vi "Validate JSON structure (LabVIEW format).vi"(8 "error in (no error)":errorcluster, 9 "Reference cluster":variant, 10 "Compare structure":string="{\r\n    \"SpecificationVersion\":\"1\",\r\n    \"CompatibleSoftwareVersions\":[\r\n        \"1.0\"\r\n    ],\r\n    \"AlgoParameters\":{\r\n        \"PartsList\":[\r\n            {\r\n                \"Name\":\"TT-1478\",\r\n                \"ImageStreams\":[\r\n                    {\r\n                        \"ThreadName\":\"TopRack\",\r\n                        \"RackEnable\":true,\r\n                        \"ThreadId\":0,\r\n                        \"RackId\":0,\r\n                        \"DifferenceParameter\":0,\r\n                        \"SplitCameraIDs\":[\r\n                            0\r\n                        ],\r\n                        \"ImagingViews\":[\r\n                            {\r\n                                \"ViewName\":\"Top\",\r\n                                \"ViewEnable\":true,\r\n                                \"ImageID\":0,\r\n                                \"CameraID\":0,\r\n                                \"CalibrationFilePath\":\"Algorithm\\\\Calibration\\\\TT Top Calib\",\r\n                                \"CalibImageFormat\":\"png\",\r\n                                \"ReferenceCoordSystem\":{\r\n                                    \"Method\":{\r\n                                        \"Algo\":\"Detect Ellipses v2\",\r\n                                        \"BaseReference\":{\r\n                                            \"OriginX\":902,\r\n                                            \"OriginY\":425,\r\n                                            \"Angle\":0,\r\n                                            \"AxisReference\":0\r\n                                        }\r\n                                    },\r\n                                    \"ROI\":[\r\n                                        {\r\n                                            \"ROI\":{\r\n                                                \"Left\":820,\r\n                                                \"Top\":170,\r\n                                                \"Right\":1110,\r\n                                                \"Bottom\":630,\r\n                                                \"Rotation\":0\r\n                                            },\r\n                                            \"EdgeOptions\":{\r\n                                                \"EdgePolarity\":2,\r\n                                                \"KernelSize\":5,\r\n                                                \"Width\":5,\r\n                                                \"MinimumEdgeStrength\":50,\r\n                                                \"InterpolationType\":0,\r\n                                                \"DataProcessingMethod\":0\r\n                                            },\r\n                                            \"LineOptions\":{\r\n                                                \"NumberofLines\":1,\r\n                                                \"Type\":0,\r\n                                                \"MinScore\":10,\r\n                                                \"MaxScore\":1000,\r\n                                                \"Orientation\":0,\r\n                                                \"AngleRange\":60,\r\n                                                \"AngleTolerance\":10,\r\n                                                \"StepSize\":15,\r\n                                                \"MinSNR\":10,\r\n                                                \"MinPoints\":25,\r\n                                                \"HoughIterations\":5\r\n                                            },\r\n                                            \"Process\":0,\r\n                                            \"StepSize\":10,\r\n                                            \"SearchDirection\":1,\r\n                                            \"CircleEdgeOptions\":{\r\n                                                \"SearchDirection\":1,\r\n                                                \"EdgeOptions\":{\r\n                                                    \"EdgePolarity\":0,\r\n                                                    \"KernelSize\":7,\r\n                                                    \"Width\":5,\r\n                                                    \"MinimumEdgeStrength\":50,\r\n                                                    \"InterpolationType\":0,\r\n                                                    \"DataProcessingMethod\":0\r\n                                                }\r\n                                            },\r\n                                            \"CircleFitOptions\":{\r\n                                                \"Process\":3,\r\n                                                \"StepSize\":3,\r\n                                                \"MAxPixelRadius\":3\r\n                                            },\r\n                                            \"CircleSearchDirection\":1,\r\n                                            \"CurveParameters\":{\r\n                                                \"ExtractionMode\":0,\r\n                                                \"EdgeThreshold\":50,\r\n                                                \"EdgeFilterSize\":0,\r\n                                                \"MinLength\":25,\r\n                                                \"RowSearchStepSize\":15,\r\n                                                \"ColSearchStepSize\":15,\r\n                                                \"MaxEndpointGap\":10,\r\n                                                \"Closed\":true,\r\n                                                \"Subpixel\":true\r\n                                            },\r\n                                            \"MinimumMatchScore\":800,\r\n                                            \"CircleDescriptor\":{\r\n                                                \"MinRadius\":3,\r\n                                                \"MaxRadius\":200\r\n                                            },\r\n                                            \"EllipseDescriptor\":{\r\n                                                \"MinMajorRadius\":3,\r\n                                                \"MaxMajorRadius\":200,\r\n                                                \"MinMinorRadius\":3,\r\n                                                \"MaxMinorRadius\":100\r\n                                            },\r\n                                            \"ParallelLines\":{\r\n                                                \"First\":30,\r\n                                                \"Second\":45,\r\n                                                \"Third\":60\r\n                                            }\r\n                                        }\r\n                                    ],\r\n                                    \"Name\":\"FirstReference\",\r\n                                    \"OverlayOptions\":{\r\n                                        \"OverlayEnable\":true,\r\n                                        \"OverlayText\":\"Height\",\r\n                                        \"OverlayCoords\":[\r\n                                            5,\r\n                                            8\r\n                                        ],\r\n                                        \"OverlayAngle\":56,\r\n                                        \"OverlayTextSize\":6,\r\n                                        \"OverlayTextColor\":\"Blue\",\r\n                                        \"OverlayROI\":false,\r\n                                        \"OverlayRakeLine\":false,\r\n                                        \"OverlayPoints\":false\r\n                                    }\r\n                                },\r\n                                \"CameraAngle\":[\r\n                                    15\r\n                                ]\r\n                            }\r\n                        ]\r\n                    }\r\n                ],\r\n                \"Measurements\":[\r\n                    {\r\n                        \"RackID\":0,\r\n                        \"ImageID\":0,\r\n                        \"CameraID\":0,\r\n                        \"MeasurementId\":1,\r\n                        \"Name\":\"L\",\r\n                        \"AlgoName\":\"AET\",\r\n                        \"Type\":\"Max\",\r\n                        \"MeasurementEnable\":true,\r\n                        \"AlgorithmSequence\":{\r\n                            \"RefernceEdge\":{\r\n                                \"Enable\":true,\r\n                                \"Method\":\"LineFinding\",\r\n                                \"RefROI\":{\r\n                                    \"Left\":330,\r\n                                    \"Top\":200,\r\n                                    \"Right\":400,\r\n                                    \"Bottom\":500,\r\n                                    \"Rotation\":0\r\n                                },\r\n                                \"EdgeOptions\":{\r\n                                    \"EdgePoarity\":2,\r\n                                    \"KernelSize\":5,\r\n                                    \"Width\":5,\r\n                                    \"MinimumEdgeStrength\":50,\r\n                                    \"InterpolationType\":0,\r\n                                    \"DataProcessingMethod\":0\r\n                                },\r\n                                \"LineOptions\":{\r\n                                    \"NumberofLines\":1,\r\n                                    \"Type\":0,\r\n                                    \"MinScore\":10,\r\n                                    \"MaxScore\":1000,\r\n                                    \"Orientation\":5,\r\n                                    \"AngleRange\":70,\r\n                                    \"AngleTolerance\":1,\r\n                                    \"StepSize\":3,\r\n                                    \"MinSNR\":0,\r\n                                    \"MinPoints\":25,\r\n                                    \"HoughIterations\":5\r\n                                },\r\n                                \"SearchDirection\":2\r\n                            },\r\n                            \"Measurement\":{\r\n                                \"ROI1\":{\r\n                                    \"Enable\":true,\r\n                                    \"ROI\":{\r\n                                        \"Left\":320,\r\n                                        \"Top\":200,\r\n                                        \"Right\":330,\r\n                                        \"Bottom\":600,\r\n                                        \"Rotation\":0\r\n                                    },\r\n                                    \"EdgeOptions\":{\r\n                                        \"EdgePoarity\":0,\r\n                                        \"KernelSize\":5,\r\n                                        \"Width\":5,\r\n                                        \"MinimumEdgeStrength\":50,\r\n                                        \"InterpolationType\":0,\r\n                                        \"DataProcessingMethod\":0\r\n                                    },\r\n                                    \"LineOptions\":{\r\n                                        \"NumberofLines\":1,\r\n                                        \"Type\":1,\r\n                                        \"MinScore\":10,\r\n                                        \"MaxScore\":1000,\r\n                                        \"Orientation\":0,\r\n                                        \"AngleRange\":30,\r\n                                        \"AngleTolerance\":1,\r\n                                        \"StepSize\":3,\r\n                                        \"MinSNR\":0,\r\n                                        \"MinPoints\":25,\r\n                                        \"HoughIterations\":5\r\n                                    },\r\n                                    \"Process\":1,\r\n                                    \"StepSize\":3,\r\n                                    \"SearchDirection\":2,\r\n                                    \"CircleEdgeOptions\":{\r\n                                        \"SearchDirection\":0,\r\n                                        \"EdgeOptions\":{\r\n                                            \"EdgePoarity\":2,\r\n                                            \"KernelSize\":5,\r\n                                            \"Width\":5,\r\n                                            \"MinimumEdgeStrength\":50,\r\n                                            \"InterpolationType\":1,\r\n                                            \"DataProcessingMethod\":1\r\n                                        }\r\n                                    },\r\n                                    \"CircleFitOptions\":{\r\n                                        \"Process\":3,\r\n                                        \"StepSize\":3,\r\n                                        \"MAxPixelRadius\":3.8500000000000000000\r\n                                    },\r\n                                    \"CircleSearchDirection\":1,\r\n                                    \"CurveParameters\":{\r\n                                        \"ExtractionMode\":0,\r\n                                        \"EdgeThreshold\":50,\r\n                                        \"EdgeFilterSize\":0,\r\n                                        \"MinLength\":25,\r\n                                        \"RowSearchStepSize\":15,\r\n                                        \"ColSearchStepSize\":15,\r\n                                        \"MaxEndpointGap\":10,\r\n                                        \"Closed\":true,\r\n                                        \"Subpixel\":true\r\n                                    },\r\n                                    \"MinimumMatchScore\":800,\r\n                                    \"CircleDescriptor\":{\r\n                                        \"MinRadius\":3,\r\n                                        \"MaxRadius\":200\r\n                                    },\r\n                                    \"EllipseDescriptor\":{\r\n                                        \"MinMajorRadius\":2,\r\n                                        \"MaxMajorRadius\":200,\r\n                                        \"MinMinorRadius\":2,\r\n                                        \"MaxMinorRadius\":100\r\n                                    }\r\n                                },\r\n                                \"ROI2\":{\r\n                                    \"Enable\":false,\r\n                                    \"ROI\":{\r\n                                        \"Left\":739,\r\n                                        \"Top\":305,\r\n                                        \"Right\":763,\r\n                                        \"Bottom\":538,\r\n                                        \"Rotation\":0\r\n                                    },\r\n                                    \"EdgeOptions\":{\r\n                                        \"EdgePoarity\":0,\r\n                                        \"KernelSize\":5,\r\n                                        \"Width\":5,\r\n                                        \"MinimumEdgeStrength\":50,\r\n                                        \"InterpolationType\":0,\r\n                                        \"DataProcessingMethod\":0\r\n                                    },\r\n                                    \"LineOptions\":{\r\n                                        \"NumberofLines\":1,\r\n                                        \"Type\":1,\r\n                                        \"MinScore\":10,\r\n                                        \"MaxScore\":1000,\r\n                                        \"Orientation\":0,\r\n                                        \"AngleRange\":30,\r\n                                        \"AngleTolerance\":1,\r\n                                        \"StepSize\":3,\r\n                                        \"MinSNR\":0,\r\n                                        \"MinPoints\":25,\r\n                                        \"HoughIterations\":5\r\n                                    },\r\n                                    \"Process\":1,\r\n                                    \"StepSize\":2,\r\n                                    \"SearchDirection\":2,\r\n                                    \"CircleEdgeOptions\":{\r\n                                        \"SearchDirection\":0,\r\n                                        \"EdgeOptions\":{\r\n                                            \"EdgePoarity\":2,\r\n                                            \"KernelSize\":3,\r\n                                            \"Width\":3,\r\n                                            \"MinimumEdgeStrength\":50,\r\n                                            \"InterpolationType\":1,\r\n                                            \"DataProcessingMethod\":1\r\n                                        }\r\n                                    },\r\n                                    \"CircleFitOptions\":{\r\n                                        \"Process\":3,\r\n                                        \"StepSize\":3,\r\n                                        \"MAxPixelRadius\":3.8500000000000000000\r\n                                    },\r\n                                    \"CircleSearchDirection\":1,\r\n                                    \"CurveParameters\":{\r\n                                        \"ExtractionMode\":0,\r\n                                        \"EdgeThreshold\":50,\r\n                                        \"EdgeFilterSize\":0,\r\n                                        \"MinLength\":25,\r\n                                        \"RowSearchStepSize\":15,\r\n                                        \"ColSearchStepSize\":15,\r\n                                        \"MaxEndpointGap\":10,\r\n                                        \"Closed\":true,\r\n                                        \"Subpixel\":true\r\n                                    },\r\n                                    \"MinimumMatchScore\":800,\r\n                                    \"CircleDescriptor\":{\r\n                                        \"MinRadius\":3,\r\n                                        \"MaxRadius\":200\r\n                                    },\r\n                                    \"EllipseDescriptor\":{\r\n                                        \"MinMajorRadius\":2,\r\n                                        \"MaxMajorRadius\":200,\r\n                                        \"MinMinorRadius\":2,\r\n                                        \"MaxMinorRadius\":100\r\n                                    }\r\n                                }\r\n                            }\r\n                        },\r\n                        \"MathExpression\":{\r\n                            \"Algorithm\":\"Default\",\r\n                            \"MathExpression\":\"c = 1*c + 0\",\r\n                            \"ResultVariable\":\"c\"\r\n                        },\r\n                        \"MathCorrectionParameters\":{\r\n                            \"Radius\":1.1000000000000000000,\r\n                            \"CurlGap\":0.90000000000000000000,\r\n                            \"Thickness\":0.32000000000000000000,\r\n                            \"MeasurementIndices\":[\r\n                                1\r\n                            ],\r\n                            \"MathAlgoName\":\"Test\",\r\n                            \"MathAlgoFormula\":\"Test2\",\r\n                            \"CorrectionForAngle\":[\r\n                                -2\r\n                            ],\r\n                            \"NumericAray\":[\r\n                                1.1000000000000000000\r\n                            ],\r\n                            \"StringArray\":[\r\n                                \"Test\"\r\n                            ]\r\n                        },\r\n                        \"ResultVariableCluster\":{\r\n                            \"RVName\":\"c\",\r\n                            \"RVSequence\":\"MeasROI1\",\r\n                            \"RVIndex\":1,\r\n                            \"RVID\":1,\r\n                            \"RVValue\":22.600000000000000000\r\n                        },\r\n                        \"CalibrationCoefficients\":{\r\n                            \"A1\":1.6800000000000000000,\r\n                            \"A2\":1.7800000000000000000,\r\n                            \"A3\":1.7600000000000000000\r\n                        },\r\n                        \"UserCalibCoefficients\":{\r\n                            \"UserCorrectionLinearityCoeff\":0.80000000000000000000,\r\n                            \"UserCorrectionBiasCoeff\":0.44300000000000000000\r\n                        },\r\n                        \"SpecValues\":{\r\n                            \"LCL\":2.1500000000000000000,\r\n                            \"UCL\":2.3500000000000000000,\r\n                            \"LSL\":2.1500000000000000000,\r\n                            \"USL\":2.3500000000000000000,\r\n                            \"NominalValue\":2.2500000000000000000\r\n                        },\r\n                        \"OverlayOptions\":{\r\n                            \"OverlayEnable\":true,\r\n                            \"OverlayText\":\"Width\",\r\n                            \"OverlayCoords\":[\r\n                                5,\r\n                                8\r\n                            ],\r\n                            \"OverlayAngle\":56,\r\n                            \"OverlayTextSize\":6,\r\n                            \"OverlayTextColor\":\"Blue\",\r\n                            \"OverlayROI\":true,\r\n                            \"OverlayRakeLine\":true,\r\n                            \"OverlayPoints\":true\r\n                        },\r\n                        \"DatalogEnable\":true,\r\n                        \"DisplayIcon\":\"C:\\\\Desktop\\\\displayimage.png\"\r\n                    }\r\n                ]\r\n            },\r\n            {\r\n                \"Name\":\"Part 3\",\r\n                \"ImageStreams\":[\r\n                    {\r\n                        \"ThreadName\":\"TopRack3\",\r\n                        \"RackEnable\":true,\r\n                        \"ThreadId\":0,\r\n                        \"RackId\":0,\r\n                        \"DifferenceParameter\":0,\r\n                        \"SplitCameraIDs\":[\r\n                            0\r\n                        ],\r\n                        \"ImagingViews\":[\r\n                            {\r\n                                \"ViewName\":\"Top2\",\r\n                                \"ViewEnable\":true,\r\n                                \"ImageID\":0,\r\n                                \"CameraID\":0,\r\n                                \"CalibrationFilePath\":\"Algorithm\\\\Calibration\\\\TT Top Calib\",\r\n                                \"CalibImageFormat\":\"png\",\r\n                                \"ReferenceCoordSystem\":{\r\n                                    \"Method\":{\r\n                                        \"Algo\":\"Detect Ellipses v2\",\r\n                                        \"BaseReference\":{\r\n                                            \"OriginX\":902,\r\n                                            \"OriginY\":425,\r\n                                            \"Angle\":0,\r\n                                            \"AxisReference\":0\r\n                                        }\r\n                                    },\r\n                                    \"ROI\":[\r\n                                        {\r\n                                            \"ROI\":{\r\n                                                \"Left\":820,\r\n                                                \"Top\":170,\r\n                                                \"Right\":1110,\r\n                                                \"Bottom\":630,\r\n                                                \"Rotation\":0\r\n                                            },\r\n                                            \"EdgeOptions\":{\r\n                                                \"EdgePolarity\":2,\r\n                                                \"KernelSize\":5,\r\n                                                \"Width\":5,\r\n                                                \"MinimumEdgeStrength\":50,\r\n                                                \"InterpolationType\":0,\r\n                                                \"DataProcessingMethod\":0\r\n                                            },\r\n                                            \"LineOptions\":{\r\n                                                \"NumberofLines\":1,\r\n                                                \"Type\":0,\r\n                                                \"MinScore\":10,\r\n                                                \"MaxScore\":1000,\r\n                                                \"Orientation\":0,\r\n                                                \"AngleRange\":60,\r\n                                                \"AngleTolerance\":10,\r\n                                                \"StepSize\":15,\r\n                                                \"MinSNR\":10,\r\n                                                \"MinPoints\":25,\r\n                                                \"HoughIterations\":5\r\n                                            },\r\n                                            \"Process\":0,\r\n                                            \"StepSize\":10,\r\n                                            \"SearchDirection\":1,\r\n                                            \"CircleEdgeOptions\":{\r\n                                                \"SearchDirection\":1,\r\n                                                \"EdgeOptions\":{\r\n                                                    \"EdgePolarity\":0,\r\n                                                    \"KernelSize\":7,\r\n                                                    \"Width\":5,\r\n                                                    \"MinimumEdgeStrength\":50,\r\n                                                    \"InterpolationType\":0,\r\n                                                    \"DataProcessingMethod\":0\r\n                                                }\r\n                                            },\r\n                                            \"CircleFitOptions\":{\r\n                                                \"Process\":3,\r\n                                                \"StepSize\":3,\r\n                                                \"MAxPixelRadius\":3\r\n                                            },\r\n                                            \"CircleSearchDirection\":1,\r\n                                            \"CurveParameters\":{\r\n                                                \"ExtractionMode\":0,\r\n                                                \"EdgeThreshold\":50,\r\n                                                \"EdgeFilterSize\":0,\r\n                                                \"MinLength\":25,\r\n                                                \"RowSearchStepSize\":15,\r\n                                                \"ColSearchStepSize\":15,\r\n                                                \"MaxEndpointGap\":10,\r\n                                                \"Closed\":true,\r\n                                                \"Subpixel\":true\r\n                                            },\r\n                                            \"MinimumMatchScore\":800,\r\n                                            \"CircleDescriptor\":{\r\n                                                \"MinRadius\":3,\r\n                                                \"MaxRadius\":200\r\n                                            },\r\n                                            \"EllipseDescriptor\":{\r\n                                                \"MinMajorRadius\":3,\r\n                                                \"MaxMajorRadius\":200,\r\n                                                \"MinMinorRadius\":3,\r\n                                                \"MaxMinorRadius\":100\r\n                                            },\r\n                                            \"ParallelLines\":{\r\n                                                \"First\":30,\r\n                                                \"Second\":45,\r\n                                                \"Third\":60\r\n                                            }\r\n                                        }\r\n                                    ],\r\n                                    \"Name\":\"FirstReference\",\r\n                                    \"OverlayOptions\":{\r\n                                        \"OverlayEnable\":true,\r\n                                        \"OverlayText\":\"Height\",\r\n                                        \"OverlayCoords\":[\r\n                                            5,\r\n                                            8\r\n                                        ],\r\n                                        \"OverlayAngle\":56,\r\n                                        \"OverlayTextSize\":6,\r\n                                        \"OverlayTextColor\":\"Blue\",\r\n                                        \"OverlayROI\":false,\r\n                                        \"OverlayRakeLine\":false,\r\n                                        \"OverlayPoints\":false\r\n                                    }\r\n                                },\r\n                                \"CameraAngle\":[\r\n                                    15\r\n                                ]\r\n                            }\r\n                        ]\r\n                    }\r\n                ],\r\n                \"Measurements\":[\r\n                    {\r\n                        \"RackID\":0,\r\n                        \"ImageID\":0,\r\n                        \"CameraID\":0,\r\n                        \"MeasurementId\":2,\r\n                        \"Name\":\"Measurement 2\",\r\n                        \"AlgoName\":\"AET\",\r\n                        \"Type\":\"Max\",\r\n                        \"MeasurementEnable\":true,\r\n                        \"AlgorithmSequence\":{\r\n                            \"RefernceEdge\":{\r\n                                \"Enable\":true,\r\n                                \"Method\":\"LineFinding\",\r\n                                \"RefROI\":{\r\n                                    \"Left\":330,\r\n                                    \"Top\":200,\r\n                                    \"Right\":400,\r\n                                    \"Bottom\":500,\r\n                                    \"Rotation\":0\r\n                                },\r\n                                \"EdgeOptions\":{\r\n                                    \"EdgePoarity\":2,\r\n                                    \"KernelSize\":5,\r\n                                    \"Width\":5,\r\n                                    \"MinimumEdgeStrength\":50,\r\n                                    \"InterpolationType\":0,\r\n                                    \"DataProcessingMethod\":0\r\n                                },\r\n                                \"LineOptions\":{\r\n                                    \"NumberofLines\":1,\r\n                                    \"Type\":0,\r\n                                    \"MinScore\":10,\r\n                                    \"MaxScore\":1000,\r\n                                    \"Orientation\":5,\r\n                                    \"AngleRange\":70,\r\n                                    \"AngleTolerance\":1,\r\n                                    \"StepSize\":3,\r\n                                    \"MinSNR\":0,\r\n                                    \"MinPoints\":25,\r\n                                    \"HoughIterations\":5\r\n                                },\r\n                                \"SearchDirection\":2\r\n                            },\r\n                            \"Measurement\":{\r\n                                \"ROI1\":{\r\n                                    \"Enable\":true,\r\n                                    \"ROI\":{\r\n                                        \"Left\":320,\r\n                                        \"Top\":200,\r\n                                        \"Right\":330,\r\n                                        \"Bottom\":600,\r\n                                        \"Rotation\":0\r\n                                    },\r\n                                    \"EdgeOptions\":{\r\n                                        \"EdgePoarity\":0,\r\n                                        \"KernelSize\":5,\r\n                                        \"Width\":5,\r\n                                        \"MinimumEdgeStrength\":50,\r\n                                        \"InterpolationType\":0,\r\n                                        \"DataProcessingMethod\":0\r\n                                    },\r\n                                    \"LineOptions\":{\r\n                                        \"NumberofLines\":1,\r\n                                        \"Type\":1,\r\n                                        \"MinScore\":10,\r\n                                        \"MaxScore\":1000,\r\n                                        \"Orientation\":0,\r\n                                        \"AngleRange\":30,\r\n                                        \"AngleTolerance\":1,\r\n                                        \"StepSize\":3,\r\n                                        \"MinSNR\":0,\r\n                                        \"MinPoints\":25,\r\n                                        \"HoughIterations\":5\r\n                                    },\r\n                                    \"Process\":1,\r\n                                    \"StepSize\":3,\r\n                                    \"SearchDirection\":2,\r\n                                    \"CircleEdgeOptions\":{\r\n                                        \"SearchDirection\":0,\r\n                                        \"EdgeOptions\":{\r\n                                            \"EdgePoarity\":2,\r\n                                            \"KernelSize\":5,\r\n                                            \"Width\":5,\r\n                                            \"MinimumEdgeStrength\":50,\r\n                                            \"InterpolationType\":1,\r\n                                            \"DataProcessingMethod\":1\r\n                                        }\r\n                                    },\r\n                                    \"CircleFitOptions\":{\r\n                                        \"Process\":3,\r\n                                        \"StepSize\":3,\r\n                                        \"MAxPixelRadius\":3.8500000000000000000\r\n                                    },\r\n                                    \"CircleSearchDirection\":1,\r\n                                    \"CurveParameters\":{\r\n                                        \"ExtractionMode\":0,\r\n                                        \"EdgeThreshold\":50,\r\n                                        \"EdgeFilterSize\":0,\r\n                                        \"MinLength\":25,\r\n                                        \"RowSearchStepSize\":15,\r\n                                        \"ColSearchStepSize\":15,\r\n                                        \"MaxEndpointGap\":10,\r\n                                        \"Closed\":true,\r\n                                        \"Subpixel\":true\r\n                                    },\r\n                                    \"MinimumMatchScore\":800,\r\n                                    \"CircleDescriptor\":{\r\n                                        \"MinRadius\":3,\r\n                                        \"MaxRadius\":200\r\n                                    },\r\n                                    \"EllipseDescriptor\":{\r\n                                        \"MinMajorRadius\":2,\r\n                                        \"MaxMajorRadius\":200,\r\n                                        \"MinMinorRadius\":2,\r\n                                        \"MaxMinorRadius\":100\r\n                                    }\r\n                                },\r\n                                \"ROI2\":{\r\n                                    \"Enable\":false,\r\n                                    \"ROI\":{\r\n                                        \"Left\":739,\r\n                                        \"Top\":305,\r\n                                        \"Right\":763,\r\n                                        \"Bottom\":538,\r\n                                        \"Rotation\":0\r\n                                    },\r\n                                    \"EdgeOptions\":{\r\n                                        \"EdgePoarity\":0,\r\n                                        \"KernelSize\":5,\r\n                                        \"Width\":5,\r\n                                        \"MinimumEdgeStrength\":50,\r\n                                        \"InterpolationType\":0,\r\n                                        \"DataProcessingMethod\":0\r\n                                    },\r\n                                    \"LineOptions\":{\r\n                                        \"NumberofLines\":1,\r\n                                        \"Type\":1,\r\n                                        \"MinScore\":10,\r\n                                        \"MaxScore\":1000,\r\n                                        \"Orientation\":0,\r\n                                        \"AngleRange\":30,\r\n                                        \"AngleTolerance\":1,\r\n                                        \"StepSize\":3,\r\n                                        \"MinSNR\":0,\r\n                                        \"MinPoints\":25,\r\n                                        \"HoughIterations\":5\r\n                                    },\r\n                                    \"Process\":1,\r\n                                    \"StepSize\":2,\r\n                                    \"SearchDirection\":2,\r\n                                    \"CircleEdgeOptions\":{\r\n                                        \"SearchDirection\":0,\r\n                                        \"EdgeOptions\":{\r\n                                            \"EdgePoarity\":2,\r\n                                            \"KernelSize\":3,\r\n                                            \"Width\":3,\r\n                                            \"MinimumEdgeStrength\":50,\r\n                                            \"InterpolationType\":1,\r\n                                            \"DataProcessingMethod\":1\r\n                                        }\r\n                                    },\r\n                                    \"CircleFitOptions\":{\r\n                                        \"Process\":3,\r\n                                        \"StepSize\":3,\r\n                                        \"MAxPixelRadius\":3.8500000000000000000\r\n                                    },\r\n                                    \"CircleSearchDirection\":1,\r\n                                    \"CurveParameters\":{\r\n                                        \"ExtractionMode\":0,\r\n                                        \"EdgeThreshold\":50,\r\n                                        \"EdgeFilterSize\":0,\r\n                                        \"MinLength\":25,\r\n                                        \"RowSearchStepSize\":15,\r\n                                        \"ColSearchStepSize\":15,\r\n                                        \"MaxEndpointGap\":10,\r\n                                        \"Closed\":true,\r\n                                        \"Subpixel\":true\r\n                                    },\r\n                                    \"MinimumMatchScore\":800,\r\n                                    \"CircleDescriptor\":{\r\n                                        \"MinRadius\":3,\r\n                                        \"MaxRadius\":200\r\n                                    },\r\n                                    \"EllipseDescriptor\":{\r\n                                        \"MinMajorRadius\":2,\r\n                                        \"MaxMajorRadius\":200,\r\n                                        \"MinMinorRadius\":2,\r\n                                        \"MaxMinorRadius\":100\r\n                                    }\r\n                                }\r\n                            }\r\n                        },\r\n                        \"MathExpression\":{\r\n                            \"Algorithm\":\"Default\",\r\n                            \"MathExpression\":\"c = 1*c + 0\",\r\n                            \"ResultVariable\":\"c\"\r\n                        },\r\n                        \"MathCorrectionParameters\":{\r\n                            \"Radius\":1.1000000000000000000,\r\n                            \"CurlGap\":0.90000000000000000000,\r\n                            \"Thickness\":0.32000000000000000000,\r\n                            \"MeasurementIndices\":[\r\n                                1\r\n                            ],\r\n                            \"MathAlgoName\":\"Test\",\r\n                            \"MathAlgoFormula\":\"Test2\",\r\n                            \"CorrectionForAngle\":[\r\n                                -2\r\n                            ],\r\n                            \"NumericAray\":[\r\n                                1.1000000000000000000\r\n                            ],\r\n                            \"StringArray\":[\r\n                                \"Test\"\r\n                            ]\r\n                        },\r\n                        \"ResultVariableCluster\":{\r\n                            \"RVName\":\"c\",\r\n                            \"RVSequence\":\"MeasROI1\",\r\n                            \"RVIndex\":1,\r\n                            \"RVID\":1,\r\n                            \"RVValue\":22.600000000000000000\r\n                        },\r\n                        \"CalibrationCoefficients\":{\r\n                            \"A1\":1.6800000000000000000,\r\n                            \"A2\":1.7800000000000000000,\r\n                            \"A3\":1.7600000000000000000\r\n                        },\r\n                        \"UserCalibCoefficients\":{\r\n                            \"UserCorrectionLinearityCoeff\":0.80000000000000000000,\r\n                            \"UserCorrectionBiasCoeff\":0.44300000000000000000\r\n                        },\r\n                        \"SpecValues\":{\r\n                            \"LCL\":2.1500000000000000000,\r\n                            \"UCL\":2.3500000000000000000,\r\n                            \"LSL\":2.1500000000000000000,\r\n                            \"USL\":2.3500000000000000000,\r\n                            \"NominalValue\":2.2500000000000000000\r\n                        },\r\n                        \"OverlayOptions\":{\r\n                            \"OverlayEnable\":true,\r\n                            \"OverlayText\":\"Width\",\r\n                            \"OverlayCoords\":[\r\n                                5,\r\n                                8\r\n                            ],\r\n                            \"OverlayAngle\":56,\r\n                            \"OverlayTextSize\":6,\r\n                            \"OverlayTextColor\":\"Blue\",\r\n                            \"OverlayROI\":true,\r\n                            \"OverlayRakeLine\":true,\r\n                            \"OverlayPoints\":true\r\n                        },\r\n                        \"DatalogEnable\":true,\r\n                        \"DisplayIcon\":\"C:\\\\Desktop\\\\displayimage.png\"\r\n                    }\r\n                ]\r\n            },\r\n            {\r\n                \"Name\":\"Part 3\",\r\n                \"ImageStreams\":[\r\n                    {\r\n                        \"ThreadName\":\"TopRack3\",\r\n                        \"RackEnable\":true,\r\n                        \"ThreadId\":0,\r\n                        \"RackId\":0,\r\n                        \"DifferenceParameter\":0,\r\n                        \"SplitCameraIDs\":[\r\n                            0\r\n                        ],\r\n                        \"ImagingViews\":[\r\n                            {\r\n                                \"ViewName\":\"Top2\",\r\n                                \"ViewEnable\":true,\r\n                                \"ImageID\":0,\r\n                                \"CameraID\":0,\r\n                                \"CalibrationFilePath\":\"Algorithm\\\\Calibration\\\\TT Top Calib\",\r\n                                \"CalibImageFormat\":\"png\",\r\n                                \"ReferenceCoordSystem\":{\r\n                                    \"Method\":{\r\n                                        \"Algo\":\"Detect Ellipses v2\",\r\n                                        \"BaseReference\":{\r\n                                            \"OriginX\":902,\r\n                                            \"OriginY\":425,\r\n                                            \"Angle\":0,\r\n                                            \"AxisReference\":0\r\n                                        }\r\n                                    },\r\n                                    \"ROI\":[\r\n                                        {\r\n                                            \"ROI\":{\r\n                                                \"Left\":820,\r\n                                                \"Top\":170,\r\n                                                \"Right\":1110,\r\n                                                \"Bottom\":630,\r\n                                                \"Rotation\":0\r\n                                            },\r\n                                            \"EdgeOptions\":{\r\n                                                \"EdgePolarity\":2,\r\n                                                \"KernelSize\":5,\r\n                                                \"Width\":5,\r\n                                                \"MinimumEdgeStrength\":50,\r\n                                                \"InterpolationType\":0,\r\n                                                \"DataProcessingMethod\":0\r\n                                            },\r\n                                            \"LineOptions\":{\r\n                                                \"NumberofLines\":1,\r\n                                                \"Type\":0,\r\n                                                \"MinScore\":10,\r\n                                                \"MaxScore\":1000,\r\n                                                \"Orientation\":0,\r\n                                                \"AngleRange\":60,\r\n                                                \"AngleTolerance\":10,\r\n                                                \"StepSize\":15,\r\n                                                \"MinSNR\":10,\r\n                                                \"MinPoints\":25,\r\n                                                \"HoughIterations\":5\r\n                                            },\r\n                                            \"Process\":0,\r\n                                            \"StepSize\":10,\r\n                                            \"SearchDirection\":1,\r\n                                            \"CircleEdgeOptions\":{\r\n                                                \"SearchDirection\":1,\r\n                                                \"EdgeOptions\":{\r\n                                                    \"EdgePolarity\":0,\r\n                                                    \"KernelSize\":7,\r\n                                                    \"Width\":5,\r\n                                                    \"MinimumEdgeStrength\":50,\r\n                                                    \"InterpolationType\":0,\r\n                                                    \"DataProcessingMethod\":0\r\n                                                }\r\n                                            },\r\n                                            \"CircleFitOptions\":{\r\n                                                \"Process\":3,\r\n                                                \"StepSize\":3,\r\n                                                \"MAxPixelRadius\":3\r\n                                            },\r\n                                            \"CircleSearchDirection\":1,\r\n                                            \"CurveParameters\":{\r\n                                                \"ExtractionMode\":0,\r\n                                                \"EdgeThreshold\":50,\r\n                                                \"EdgeFilterSize\":0,\r\n                                                \"MinLength\":25,\r\n                                                \"RowSearchStepSize\":15,\r\n                                                \"ColSearchStepSize\":15,\r\n                                                \"MaxEndpointGap\":10,\r\n                                                \"Closed\":true,\r\n                                                \"Subpixel\":true\r\n                                            },\r\n                                            \"MinimumMatchScore\":800,\r\n                                            \"CircleDescriptor\":{\r\n                                                \"MinRadius\":3,\r\n                                                \"MaxRadius\":200\r\n                                            },\r\n                                            \"EllipseDescriptor\":{\r\n                                                \"MinMajorRadius\":3,\r\n                                                \"MaxMajorRadius\":200,\r\n                                                \"MinMinorRadius\":3,\r\n                                                \"MaxMinorRadius\":100\r\n                                            },\r\n                                            \"ParallelLines\":{\r\n                                                \"First\":30,\r\n                                                \"Second\":45,\r\n                                                \"Third\":60\r\n                                            }\r\n                                        }\r\n                                    ],\r\n                                    \"Name\":\"FirstReference\",\r\n                                    \"OverlayOptions\":{\r\n                                        \"OverlayEnable\":true,\r\n                                        \"OverlayText\":\"Height\",\r\n                                        \"OverlayCoords\":[\r\n                                            5,\r\n                                            8\r\n                                        ],\r\n                                        \"OverlayAngle\":56,\r\n                                        \"OverlayTextSize\":6,\r\n                                        \"OverlayTextColor\":\"Blue\",\r\n                                        \"OverlayROI\":false,\r\n                                        \"OverlayRakeLine\":false,\r\n                                        \"OverlayPoints\":false\r\n                                    }\r\n                                },\r\n                                \"CameraAngle\":[\r\n                                    15\r\n                                ]\r\n                            }\r\n                        ]\r\n                    }\r\n                ],\r\n                \"Measurements\":[\r\n                    {\r\n                        \"RackID\":0,\r\n                        \"ImageID\":0,\r\n                        \"CameraID\":0,\r\n                        \"MeasurementId\":2,\r\n                        \"Name\":\"Measurement 2\",\r\n                        \"AlgoName\":\"AET\",\r\n                        \"Type\":\"Max\",\r\n                        \"MeasurementEnable\":true,\r\n                        \"AlgorithmSequence\":{\r\n                            \"RefernceEdge\":{\r\n                                \"Enable\":true,\r\n                                \"Method\":\"LineFinding\",\r\n                                \"RefROI\":{\r\n                                    \"Left\":330,\r\n                                    \"Top\":200,\r\n                                    \"Right\":400,\r\n                                    \"Bottom\":500,\r\n                                    \"Rotation\":0\r\n                                },\r\n                                \"EdgeOptions\":{\r\n                                    \"EdgePoarity\":2,\r\n                                    \"KernelSize\":5,\r\n                                    \"Width\":5,\r\n                                    \"MinimumEdgeStrength\":50,\r\n                                    \"InterpolationType\":0,\r\n                                    \"DataProcessingMethod\":0\r\n                                },\r\n                                \"LineOptions\":{\r\n                                    \"NumberofLines\":1,\r\n                                    \"Type\":0,\r\n                                    \"MinScore\":10,\r\n                                    \"MaxScore\":1000,\r\n                                    \"Orientation\":5,\r\n                                    \"AngleRange\":70,\r\n                                    \"AngleTolerance\":1,\r\n                                    \"StepSize\":3,\r\n                                    \"MinSNR\":0,\r\n                                    \"MinPoints\":25,\r\n                                    \"HoughIterations\":5\r\n                                },\r\n                                \"SearchDirection\":2\r\n                            },\r\n                            \"Measurement\":{\r\n                                \"ROI1\":{\r\n                                    \"Enable\":true,\r\n                                    \"ROI\":{\r\n                                        \"Left\":320,\r\n                                        \"Top\":200,\r\n                                        \"Right\":330,\r\n                                        \"Bottom\":600,\r\n                                        \"Rotation\":0\r\n                                    },\r\n                                    \"EdgeOptions\":{\r\n                                        \"EdgePoarity\":0,\r\n                                        \"KernelSize\":5,\r\n                                        \"Width\":5,\r\n                                        \"MinimumEdgeStrength\":50,\r\n                                        \"InterpolationType\":0,\r\n                                        \"DataProcessingMethod\":0\r\n                                    },\r\n                                    \"LineOptions\":{\r\n                                        \"NumberofLines\":1,\r\n                                        \"Type\":1,\r\n                                        \"MinScore\":10,\r\n                                        \"MaxScore\":1000,\r\n                                        \"Orientation\":0,\r\n                                        \"AngleRange\":30,\r\n                                        \"AngleTolerance\":1,\r\n                                        \"StepSize\":3,\r\n                                        \"MinSNR\":0,\r\n                                        \"MinPoints\":25,\r\n                                        \"HoughIterations\":5\r\n                                    },\r\n                                    \"Process\":1,\r\n                                    \"StepSize\":3,\r\n                                    \"SearchDirection\":2,\r\n                                    \"CircleEdgeOptions\":{\r\n                                        \"SearchDirection\":0,\r\n                                        \"EdgeOptions\":{\r\n                                            \"EdgePoarity\":2,\r\n                                            \"KernelSize\":5,\r\n                                            \"Width\":5,\r\n                                            \"MinimumEdgeStrength\":50,\r\n                                            \"InterpolationType\":1,\r\n                                            \"DataProcessingMethod\":1\r\n                                        }\r\n                                    },\r\n                                    \"CircleFitOptions\":{\r\n                                        \"Process\":3,\r\n                                        \"StepSize\":3,\r\n                                        \"MAxPixelRadius\":3.8500000000000000000\r\n                                    },\r\n                                    \"CircleSearchDirection\":1,\r\n                                    \"CurveParameters\":{\r\n                                        \"ExtractionMode\":0,\r\n                                        \"EdgeThreshold\":50,\r\n                                        \"EdgeFilterSize\":0,\r\n                                        \"MinLength\":25,\r\n                                        \"RowSearchStepSize\":15,\r\n                                        \"ColSearchStepSize\":15,\r\n                                        \"MaxEndpointGap\":10,\r\n                                        \"Closed\":true,\r\n                                        \"Subpixel\":true\r\n                                    },\r\n                                    \"MinimumMatchScore\":800,\r\n                                    \"CircleDescriptor\":{\r\n                                        \"MinRadius\":3,\r\n                                        \"MaxRadius\":200\r\n                                    },\r\n                                    \"EllipseDescriptor\":{\r\n                                        \"MinMajorRadius\":2,\r\n                                        \"MaxMajorRadius\":200,\r\n                                        \"MinMinorRadius\":2,\r\n                                        \"MaxMinorRadius\":100\r\n                                    }\r\n                                },\r\n                                \"ROI2\":{\r\n                                    \"Enable\":false,\r\n                                    \"ROI\":{\r\n                                        \"Left\":739,\r\n                                        \"Top\":305,\r\n                                        \"Right\":763,\r\n                                        \"Bottom\":538,\r\n                                        \"Rotation\":0\r\n                                    },\r\n                                    \"EdgeOptions\":{\r\n                                        \"EdgePoarity\":0,\r\n                                        \"KernelSize\":5,\r\n                                        \"Width\":5,\r\n                                        \"MinimumEdgeStrength\":50,\r\n                                        \"InterpolationType\":0,\r\n                                        \"DataProcessingMethod\":0\r\n                                    },\r\n                                    \"LineOptions\":{\r\n                                        \"NumberofLines\":1,\r\n                                        \"Type\":1,\r\n                                        \"MinScore\":10,\r\n                                        \"MaxScore\":1000,\r\n                                        \"Orientation\":0,\r\n                                        \"AngleRange\":30,\r\n                                        \"AngleTolerance\":1,\r\n                                        \"StepSize\":3,\r\n                                        \"MinSNR\":0,\r\n                                        \"MinPoints\":25,\r\n                                        \"HoughIterations\":5\r\n                                    },\r\n                                    \"Process\":1,\r\n                                    \"StepSize\":2,\r\n                                    \"SearchDirection\":2,\r\n                                    \"CircleEdgeOptions\":{\r\n                                        \"SearchDirection\":0,\r\n                                        \"EdgeOptions\":{\r\n                                            \"EdgePoarity\":2,\r\n                                            \"KernelSize\":3,\r\n                                            \"Width\":3,\r\n                                            \"MinimumEdgeStrength\":50,\r\n                                            \"InterpolationType\":1,\r\n                                            \"DataProcessingMethod\":1\r\n                                        }\r\n                                    },\r\n                                    \"CircleFitOptions\":{\r\n                                        \"Process\":3,\r\n                                        \"StepSize\":3,\r\n                                        \"MAxPixelRadius\":3.8500000000000000000\r\n                                    },\r\n                                    \"CircleSearchDirection\":1,\r\n                                    \"CurveParameters\":{\r\n                                        \"ExtractionMode\":0,\r\n                                        \"EdgeThreshold\":50,\r\n                                        \"EdgeFilterSize\":0,\r\n                                        \"MinLength\":25,\r\n                                        \"RowSearchStepSize\":15,\r\n                                        \"ColSearchStepSize\":15,\r\n                                        \"MaxEndpointGap\":10,\r\n                                        \"Closed\":true,\r\n                                        \"Subpixel\":true\r\n                                    },\r\n                                    \"MinimumMatchScore\":800,\r\n                                    \"CircleDescriptor\":{\r\n                                        \"MinRadius\":3,\r\n                                        \"MaxRadius\":200\r\n                                    },\r\n                                    \"EllipseDescriptor\":{\r\n                                        \"MinMajorRadius\":2,\r\n                                        \"MaxMajorRadius\":200,\r\n                                        \"MinMinorRadius\":2,\r\n                                        \"MaxMinorRadius\":100\r\n                                    }\r\n                                }\r\n                            }\r\n                        },\r\n                        \"MathExpression\":{\r\n                            \"Algorithm\":\"Default\",\r\n                            \"MathExpression\":\"c = 1*c + 0\",\r\n                            \"ResultVariable\":\"c\"\r\n                        },\r\n                        \"MathCorrectionParameters\":{\r\n                            \"Radius\":1.1000000000000000000,\r\n                            \"CurlGap\":0.90000000000000000000,\r\n                            \"Thickness\":0.32000000000000000000,\r\n                            \"MeasurementIndices\":[\r\n                                1\r\n                            ],\r\n                            \"MathAlgoName\":\"Test\",\r\n                            \"MathAlgoFormula\":\"Test2\",\r\n                            \"CorrectionForAngle\":[\r\n                                -2\r\n                            ],\r\n                            \"NumericAray\":[\r\n                                1.1000000000000000000\r\n                            ],\r\n                            \"StringArray\":[\r\n                                \"Test\"\r\n                            ]\r\n                        },\r\n                        \"ResultVariableCluster\":{\r\n                            \"RVName\":\"c\",\r\n                            \"RVSequence\":\"MeasROI1\",\r\n                            \"RVIndex\":1,\r\n                            \"RVID\":1,\r\n                            \"RVValue\":22.600000000000000000\r\n                        },\r\n                        \"CalibrationCoefficients\":{\r\n                            \"A1\":1.6800000000000000000,\r\n                            \"A2\":1.7800000000000000000,\r\n                            \"A3\":1.7600000000000000000\r\n                        },\r\n                        \"UserCalibCoefficients\":{\r\n                            \"UserCorrectionLinearityCoeff\":0.80000000000000000000,\r\n                            \"UserCorrectionBiasCoeff\":0.44300000000000000000\r\n                        },\r\n                        \"SpecValues\":{\r\n                            \"LCL\":2.1500000000000000000,\r\n                            \"UCL\":2.3500000000000000000,\r\n                            \"LSL\":2.1500000000000000000,\r\n                            \"USL\":2.3500000000000000000,\r\n                            \"NominalValue\":2.2500000000000000000\r\n                        },\r\n                        \"OverlayOptions\":{\r\n                            \"OverlayEnable\":true,\r\n                            \"OverlayText\":\"Width\",\r\n                            \"OverlayCoords\":[\r\n                                5,\r\n                                8\r\n                            ],\r\n                            \"OverlayAngle\":56,\r\n                            \"OverlayTextSize\":6,\r\n                            \"OverlayTextColor\":\"Blue\",\r\n                            \"OverlayROI\":true,\r\n                            \"OverlayRakeLine\":true,\r\n                            \"OverlayPoints\":true\r\n                        },\r\n                        \"DatalogEnable\":true,\r\n                        \"DisplayIcon\":\"C:\\\\Desktop\\\\displayimage.png\"\r\n                    }\r\n                ]\r\n            },\r\n            {\r\n                \"Name\":\"Part 2\",\r\n                \"ImageStreams\":[\r\n                    {\r\n                        \"ThreadName\":\"TopRack2\",\r\n                        \"RackEnable\":true,\r\n                        \"ThreadId\":0,\r\n                        \"RackId\":0,\r\n                        \"DifferenceParameter\":0,\r\n                        \"SplitCameraIDs\":[\r\n                            0\r\n                        ],\r\n                        \"ImagingViews\":[\r\n                            {\r\n                                \"ViewName\":\"Top2\",\r\n                                \"ViewEnable\":true,\r\n                                \"ImageID\":0,\r\n                                \"CameraID\":0,\r\n                                \"CalibrationFilePath\":\"Algorithm\\\\Calibration\\\\TT Top Calib\",\r\n                                \"CalibImageFormat\":\"png\",\r\n                                \"ReferenceCoordSystem\":{\r\n                                    \"Method\":{\r\n                                        \"Algo\":\"Detect Ellipses v2\",\r\n                                        \"BaseReference\":{\r\n                                            \"OriginX\":902,\r\n                                            \"OriginY\":425,\r\n                                            \"Angle\":0,\r\n                                            \"AxisReference\":0\r\n                                        }\r\n                                    },\r\n                                    \"ROI\":[\r\n                                        {\r\n                                            \"ROI\":{\r\n                                                \"Left\":820,\r\n                                                \"Top\":170,\r\n                                                \"Right\":1110,\r\n                                                \"Bottom\":630,\r\n                                                \"Rotation\":0\r\n                                            },\r\n                                            \"EdgeOptions\":{\r\n                                                \"EdgePolarity\":2,\r\n                                                \"KernelSize\":5,\r\n                                                \"Width\":5,\r\n                                                \"MinimumEdgeStrength\":50,\r\n                                                \"InterpolationType\":0,\r\n                                                \"DataProcessingMethod\":0\r\n                                            },\r\n                                            \"LineOptions\":{\r\n                                                \"NumberofLines\":1,\r\n                                                \"Type\":0,\r\n                                                \"MinScore\":10,\r\n                                                \"MaxScore\":1000,\r\n                                                \"Orientation\":0,\r\n                                                \"AngleRange\":60,\r\n                                                \"AngleTolerance\":10,\r\n                                                \"StepSize\":15,\r\n                                                \"MinSNR\":10,\r\n                                                \"MinPoints\":25,\r\n                                                \"HoughIterations\":5\r\n                                            },\r\n                                            \"Process\":0,\r\n                                            \"StepSize\":10,\r\n                                            \"SearchDirection\":1,\r\n                                            \"CircleEdgeOptions\":{\r\n                                                \"SearchDirection\":1,\r\n                                                \"EdgeOptions\":{\r\n                                                    \"EdgePolarity\":0,\r\n                                                    \"KernelSize\":7,\r\n                                                    \"Width\":5,\r\n                                                    \"MinimumEdgeStrength\":50,\r\n                                                    \"InterpolationType\":0,\r\n                                                    \"DataProcessingMethod\":0\r\n                                                }\r\n                                            },\r\n                                            \"CircleFitOptions\":{\r\n                                                \"Process\":3,\r\n                                                \"StepSize\":3,\r\n                                                \"MAxPixelRadius\":3\r\n                                            },\r\n                                            \"CircleSearchDirection\":1,\r\n                                            \"CurveParameters\":{\r\n                                                \"ExtractionMode\":0,\r\n                                                \"EdgeThreshold\":50,\r\n                                                \"EdgeFilterSize\":0,\r\n                                                \"MinLength\":25,\r\n                                                \"RowSearchStepSize\":15,\r\n                                                \"ColSearchStepSize\":15,\r\n                                                \"MaxEndpointGap\":10,\r\n                                                \"Closed\":true,\r\n                                                \"Subpixel\":true\r\n                                            },\r\n                                            \"MinimumMatchScore\":800,\r\n                                            \"CircleDescriptor\":{\r\n                                                \"MinRadius\":3,\r\n                                                \"MaxRadius\":200\r\n                                            },\r\n                                            \"EllipseDescriptor\":{\r\n                                                \"MinMajorRadius\":3,\r\n                                                \"MaxMajorRadius\":200,\r\n                                                \"MinMinorRadius\":3,\r\n                                                \"MaxMinorRadius\":100\r\n                                            },\r\n                                            \"ParallelLines\":{\r\n                                                \"First\":30,\r\n                                                \"Second\":45,\r\n                                                \"Third\":60\r\n                                            }\r\n                                        }\r\n                                    ],\r\n                                    \"Name\":\"FirstReference\",\r\n                                    \"OverlayOptions\":{\r\n                                        \"OverlayEnable\":true,\r\n                                        \"OverlayText\":\"Height\",\r\n                                        \"OverlayCoords\":[\r\n                                            5,\r\n                                            8\r\n                                        ],\r\n                                        \"OverlayAngle\":56,\r\n                                        \"OverlayTextSize\":6,\r\n                                        \"OverlayTextColor\":\"Blue\",\r\n                                        \"OverlayROI\":false,\r\n                                        \"OverlayRakeLine\":false,\r\n                                        \"OverlayPoints\":false\r\n                                    }\r\n                                },\r\n                                \"CameraAngle\":[\r\n                                    15\r\n                                ]\r\n                            }\r\n                        ]\r\n                    }\r\n                ],\r\n                \"Measurements\":[\r\n                    {\r\n                        \"RackID\":0,\r\n                        \"ImageID\":0,\r\n                        \"CameraID\":0,\r\n                        \"MeasurementId\":1,\r\n                        \"Name\":\"Measurement 2\",\r\n                        \"AlgoName\":\"AET\",\r\n                        \"Type\":\"Max\",\r\n                        \"MeasurementEnable\":true,\r\n                        \"AlgorithmSequence\":{\r\n                            \"RefernceEdge\":{\r\n                                \"Enable\":true,\r\n                                \"Method\":\"LineFinding\",\r\n                                \"RefROI\":{\r\n                                    \"Left\":330,\r\n                                    \"Top\":200,\r\n                                    \"Right\":400,\r\n                                    \"Bottom\":500,\r\n                                    \"Rotation\":0\r\n                                },\r\n                                \"EdgeOptions\":{\r\n                                    \"EdgePoarity\":2,\r\n                                    \"KernelSize\":5,\r\n                                    \"Width\":5,\r\n                                    \"MinimumEdgeStrength\":50,\r\n                                    \"InterpolationType\":0,\r\n                                    \"DataProcessingMethod\":0\r\n                                },\r\n                                \"LineOptions\":{\r\n                                    \"NumberofLines\":1,\r\n                                    \"Type\":0,\r\n                                    \"MinScore\":10,\r\n                                    \"MaxScore\":1000,\r\n                                    \"Orientation\":5,\r\n                                    \"AngleRange\":70,\r\n                                    \"AngleTolerance\":1,\r\n                                    \"StepSize\":3,\r\n                                    \"MinSNR\":0,\r\n                                    \"MinPoints\":25,\r\n                                    \"HoughIterations\":5\r\n                                },\r\n                                \"SearchDirection\":2\r\n                            },\r\n                            \"Measurement\":{\r\n                                \"ROI1\":{\r\n                                    \"Enable\":true,\r\n                                    \"ROI\":{\r\n                                        \"Left\":320,\r\n                                        \"Top\":200,\r\n                                        \"Right\":330,\r\n                                        \"Bottom\":600,\r\n                                        \"Rotation\":0\r\n                                    },\r\n                                    \"EdgeOptions\":{\r\n                                        \"EdgePoarity\":0,\r\n                                        \"KernelSize\":5,\r\n                                        \"Width\":5,\r\n                                        \"MinimumEdgeStrength\":50,\r\n                                        \"InterpolationType\":0,\r\n                                        \"DataProcessingMethod\":0\r\n                                    },\r\n                                    \"LineOptions\":{\r\n                                        \"NumberofLines\":1,\r\n                                        \"Type\":1,\r\n                                        \"MinScore\":10,\r\n                                        \"MaxScore\":1000,\r\n                                        \"Orientation\":0,\r\n                                        \"AngleRange\":30,\r\n                                        \"AngleTolerance\":1,\r\n                                        \"StepSize\":3,\r\n                                        \"MinSNR\":0,\r\n                                        \"MinPoints\":25,\r\n                                        \"HoughIterations\":5\r\n                                    },\r\n                                    \"Process\":1,\r\n                                    \"StepSize\":3,\r\n                                    \"SearchDirection\":2,\r\n                                    \"CircleEdgeOptions\":{\r\n                                        \"SearchDirection\":0,\r\n                                        \"EdgeOptions\":{\r\n                                            \"EdgePoarity\":2,\r\n                                            \"KernelSize\":5,\r\n                                            \"Width\":5,\r\n                                            \"MinimumEdgeStrength\":50,\r\n                                            \"InterpolationType\":1,\r\n                                            \"DataProcessingMethod\":1\r\n                                        }\r\n                                    },\r\n                                    \"CircleFitOptions\":{\r\n                                        \"Process\":3,\r\n                                        \"StepSize\":3,\r\n                                        \"MAxPixelRadius\":3.8500000000000000000\r\n                                    },\r\n                                    \"CircleSearchDirection\":1,\r\n                                    \"CurveParameters\":{\r\n                                        \"ExtractionMode\":0,\r\n                                        \"EdgeThreshold\":50,\r\n                                        \"EdgeFilterSize\":0,\r\n                                        \"MinLength\":25,\r\n                                        \"RowSearchStepSize\":15,\r\n                                        \"ColSearchStepSize\":15,\r\n                                        \"MaxEndpointGap\":10,\r\n                                        \"Closed\":true,\r\n                                        \"Subpixel\":true\r\n                                    },\r\n                                    \"MinimumMatchScore\":800,\r\n                                    \"CircleDescriptor\":{\r\n                                        \"MinRadius\":3,\r\n                                        \"MaxRadius\":200\r\n                                    },\r\n                                    \"EllipseDescriptor\":{\r\n                                        \"MinMajorRadius\":2,\r\n                                        \"MaxMajorRadius\":200,\r\n                                        \"MinMinorRadius\":2,\r\n                                        \"MaxMinorRadius\":100\r\n                                    }\r\n                                },\r\n                                \"ROI2\":{\r\n                                    \"Enable\":false,\r\n                                    \"ROI\":{\r\n                                        \"Left\":739,\r\n                                        \"Top\":305,\r\n                                        \"Right\":763,\r\n                                        \"Bottom\":538,\r\n                                        \"Rotation\":0\r\n                                    },\r\n                                    \"EdgeOptions\":{\r\n                                        \"EdgePoarity\":0,\r\n                                        \"KernelSize\":5,\r\n                                        \"Width\":5,\r\n                                        \"MinimumEdgeStrength\":50,\r\n                                        \"InterpolationType\":0,\r\n                                        \"DataProcessingMethod\":0\r\n                                    },\r\n                                    \"LineOptions\":{\r\n                                        \"NumberofLines\":1,\r\n                                        \"Type\":1,\r\n                                        \"MinScore\":10,\r\n                                        \"MaxScore\":1000,\r\n                                        \"Orientation\":0,\r\n                                        \"AngleRange\":30,\r\n                                        \"AngleTolerance\":1,\r\n                                        \"StepSize\":3,\r\n                                        \"MinSNR\":0,\r\n                                        \"MinPoints\":25,\r\n                                        \"HoughIterations\":5\r\n                                    },\r\n                                    \"Process\":1,\r\n                                    \"StepSize\":2,\r\n                                    \"SearchDirection\":2,\r\n                                    \"CircleEdgeOptions\":{\r\n                                        \"SearchDirection\":0,\r\n                                        \"EdgeOptions\":{\r\n                                            \"EdgePoarity\":2,\r\n                                            \"KernelSize\":3,\r\n                                            \"Width\":3,\r\n                                            \"MinimumEdgeStrength\":50,\r\n                                            \"InterpolationType\":1,\r\n                                            \"DataProcessingMethod\":1\r\n                                        }\r\n                                    },\r\n                                    \"CircleFitOptions\":{\r\n                                        \"Process\":3,\r\n                                        \"StepSize\":3,\r\n                                        \"MAxPixelRadius\":3.8500000000000000000\r\n                                    },\r\n                                    \"CircleSearchDirection\":1,\r\n                                    \"CurveParameters\":{\r\n                                        \"ExtractionMode\":0,\r\n                                        \"EdgeThreshold\":50,\r\n                                        \"EdgeFilterSize\":0,\r\n                                        \"MinLength\":25,\r\n                                        \"RowSearchStepSize\":15,\r\n                                        \"ColSearchStepSize\":15,\r\n                                        \"MaxEndpointGap\":10,\r\n                                        \"Closed\":true,\r\n                                        \"Subpixel\":true\r\n                                    },\r\n                                    \"MinimumMatchScore\":800,\r\n                                    \"CircleDescriptor\":{\r\n                                        \"MinRadius\":3,\r\n                                        \"MaxRadius\":200\r\n                                    },\r\n                                    \"EllipseDescriptor\":{\r\n                                        \"MinMajorRadius\":2,\r\n                                        \"MaxMajorRadius\":200,\r\n                                        \"MinMinorRadius\":2,\r\n                                        \"MaxMinorRadius\":100\r\n                                    }\r\n                                }\r\n                            }\r\n                        },\r\n                        \"MathExpression\":{\r\n                            \"Algorithm\":\"Default\",\r\n                            \"MathExpression\":\"c = 1*c + 0\",\r\n                            \"ResultVariable\":\"c\"\r\n                        },\r\n                        \"MathCorrectionParameters\":{\r\n                            \"Radius\":1.1000000000000000000,\r\n                            \"CurlGap\":0.90000000000000000000,\r\n                            \"Thickness\":0.32000000000000000000,\r\n                            \"MeasurementIndices\":[\r\n                                1\r\n                            ],\r\n                            \"MathAlgoName\":\"Test\",\r\n                            \"MathAlgoFormula\":\"Test2\",\r\n                            \"CorrectionForAngle\":[\r\n                                -2\r\n                            ],\r\n                            \"NumericAray\":[\r\n                                1.1000000000000000000\r\n                            ],\r\n                            \"StringArray\":[\r\n                                \"Test\"\r\n                            ]\r\n                        },\r\n                        \"ResultVariableCluster\":{\r\n                            \"RVName\":\"c\",\r\n                            \"RVSequence\":\"MeasROI1\",\r\n                            \"RVIndex\":1,\r\n                            \"RVID\":1,\r\n                            \"RVValue\":22.600000000000000000\r\n                        },\r\n                        \"CalibrationCoefficients\":{\r\n                            \"A1\":1.6800000000000000000,\r\n                            \"A2\":1.7800000000000000000,\r\n                            \"A3\":1.7600000000000000000\r\n                        },\r\n                        \"UserCalibCoefficients\":{\r\n                            \"UserCorrectionLinearityCoeff\":0.80000000000000000000,\r\n                            \"UserCorrectionBiasCoeff\":0.44300000000000000000\r\n                        },\r\n                        \"SpecValues\":{\r\n                            \"LCL\":2.1500000000000000000,\r\n                            \"UCL\":2.3500000000000000000,\r\n                            \"LSL\":2.1500000000000000000,\r\n                            \"USL\":2.3500000000000000000,\r\n                            \"NominalValue\":2.2500000000000000000\r\n                        },\r\n                        \"OverlayOptions\":{\r\n                            \"OverlayEnable\":true,\r\n                            \"OverlayText\":\"Width\",\r\n                            \"OverlayCoords\":[\r\n                                5,\r\n                                8\r\n                            ],\r\n                            \"OverlayAngle\":56,\r\n                            \"OverlayTextSize\":6,\r\n                            \"OverlayTextColor\":\"Blue\",\r\n                            \"OverlayROI\":true,\r\n                            \"OverlayRakeLine\":true,\r\n                            \"OverlayPoints\":true\r\n                        },\r\n                        \"DatalogEnable\":true,\r\n                        \"DisplayIcon\":\"C:\\\\Desktop\\\\displayimage.png\"\r\n                    }\r\n                ]\r\n            },\r\n            {\r\n                \"Name\":\"Part 1\",\r\n                \"ImageStreams\":[\r\n                    {\r\n                        \"ThreadName\":\"TopRack1\",\r\n                        \"RackEnable\":true,\r\n                        \"ThreadId\":0,\r\n                        \"RackId\":0,\r\n                        \"DifferenceParameter\":0,\r\n                        \"SplitCameraIDs\":[\r\n                            0\r\n                        ],\r\n                        \"ImagingViews\":[\r\n                            {\r\n                                \"ViewName\":\"Top1\",\r\n                                \"ViewEnable\":true,\r\n                                \"ImageID\":0,\r\n                                \"CameraID\":0,\r\n                                \"CalibrationFilePath\":\"Algorithm\\\\Calibration\\\\TT Top Calib\",\r\n                                \"CalibImageFormat\":\"png\",\r\n                                \"ReferenceCoordSystem\":{\r\n                                    \"Method\":{\r\n                                        \"Algo\":\"Detect Ellipses v2\",\r\n                                        \"BaseReference\":{\r\n                                            \"OriginX\":902,\r\n                                            \"OriginY\":425,\r\n                                            \"Angle\":0,\r\n                                            \"AxisReference\":0\r\n                                        }\r\n                                    },\r\n                                    \"ROI\":[\r\n                                        {\r\n                                            \"ROI\":{\r\n                                                \"Left\":820,\r\n                                                \"Top\":170,\r\n                                                \"Right\":1110,\r\n                                                \"Bottom\":630,\r\n                                                \"Rotation\":0\r\n                                            },\r\n                                            \"EdgeOptions\":{\r\n                                                \"EdgePolarity\":2,\r\n                                                \"KernelSize\":5,\r\n                                                \"Width\":5,\r\n                                                \"MinimumEdgeStrength\":50,\r\n                                                \"InterpolationType\":0,\r\n                                                \"DataProcessingMethod\":0\r\n                                            },\r\n                                            \"LineOptions\":{\r\n                                                \"NumberofLines\":1,\r\n                                                \"Type\":0,\r\n                                                \"MinScore\":10,\r\n                                                \"MaxScore\":1000,\r\n                                                \"Orientation\":0,\r\n                                                \"AngleRange\":60,\r\n                                                \"AngleTolerance\":10,\r\n                                                \"StepSize\":15,\r\n                                                \"MinSNR\":10,\r\n                                                \"MinPoints\":25,\r\n                                                \"HoughIterations\":5\r\n                                            },\r\n                                            \"Process\":0,\r\n                                            \"StepSize\":10,\r\n                                            \"SearchDirection\":1,\r\n                                            \"CircleEdgeOptions\":{\r\n                                                \"SearchDirection\":1,\r\n                                                \"EdgeOptions\":{\r\n                                                    \"EdgePolarity\":0,\r\n                                                    \"KernelSize\":7,\r\n                                                    \"Width\":5,\r\n                                                    \"MinimumEdgeStrength\":50,\r\n                                                    \"InterpolationType\":0,\r\n                                                    \"DataProcessingMethod\":0\r\n                                                }\r\n                                            },\r\n                                            \"CircleFitOptions\":{\r\n                                                \"Process\":3,\r\n                                                \"StepSize\":3,\r\n                                                \"MAxPixelRadius\":3\r\n                                            },\r\n                                            \"CircleSearchDirection\":1,\r\n                                            \"CurveParameters\":{\r\n                                                \"ExtractionMode\":0,\r\n                                                \"EdgeThreshold\":50,\r\n                                                \"EdgeFilterSize\":0,\r\n                                                \"MinLength\":25,\r\n                                                \"RowSearchStepSize\":15,\r\n                                                \"ColSearchStepSize\":15,\r\n                                                \"MaxEndpointGap\":10,\r\n                                                \"Closed\":true,\r\n                                                \"Subpixel\":true\r\n                                            },\r\n                                            \"MinimumMatchScore\":800,\r\n                                            \"CircleDescriptor\":{\r\n                                                \"MinRadius\":3,\r\n                                                \"MaxRadius\":200\r\n                                            },\r\n                                            \"EllipseDescriptor\":{\r\n                                                \"MinMajorRadius\":3,\r\n                                                \"MaxMajorRadius\":200,\r\n                                                \"MinMinorRadius\":3,\r\n                                                \"MaxMinorRadius\":100\r\n                                            },\r\n                                            \"ParallelLines\":{\r\n                                                \"First\":30,\r\n                                                \"Second\":45,\r\n                                                \"Third\":60\r\n                                            }\r\n                                        }\r\n                                    ],\r\n                                    \"Name\":\"FirstReference\",\r\n                                    \"OverlayOptions\":{\r\n                                        \"OverlayEnable\":true,\r\n                                        \"OverlayText\":\"Height\",\r\n                                        \"OverlayCoords\":[\r\n                                            5,\r\n                                            8\r\n                                        ],\r\n                                        \"OverlayAngle\":56,\r\n                                        \"OverlayTextSize\":6,\r\n                                        \"OverlayTextColor\":\"Blue\",\r\n                                        \"OverlayROI\":false,\r\n                                        \"OverlayRakeLine\":false,\r\n                                        \"OverlayPoints\":false\r\n                                    }\r\n                                },\r\n                                \"CameraAngle\":[\r\n                                    15\r\n                                ]\r\n                            }\r\n                        ]\r\n                    }\r\n                ],\r\n                \"Measurements\":[\r\n                    {\r\n                        \"RackID\":0,\r\n                        \"ImageID\":0,\r\n                        \"CameraID\":0,\r\n                        \"MeasurementId\":1,\r\n                        \"Name\":\"L\",\r\n                        \"AlgoName\":\"AET\",\r\n                        \"Type\":\"Max\",\r\n                        \"MeasurementEnable\":true,\r\n                        \"AlgorithmSequence\":{\r\n                            \"RefernceEdge\":{\r\n                                \"Enable\":true,\r\n                                \"Method\":\"LineFinding\",\r\n                                \"RefROI\":{\r\n                                    \"Left\":330,\r\n                                    \"Top\":200,\r\n                                    \"Right\":400,\r\n                                    \"Bottom\":500,\r\n                                    \"Rotation\":0\r\n                                },\r\n                                \"EdgeOptions\":{\r\n                                    \"EdgePoarity\":2,\r\n                                    \"KernelSize\":5,\r\n                                    \"Width\":5,\r\n                                    \"MinimumEdgeStrength\":50,\r\n                                    \"InterpolationType\":0,\r\n                                    \"DataProcessingMethod\":0\r\n                                },\r\n                                \"LineOptions\":{\r\n                                    \"NumberofLines\":1,\r\n                                    \"Type\":0,\r\n                                    \"MinScore\":10,\r\n                                    \"MaxScore\":1000,\r\n                                    \"Orientation\":5,\r\n                                    \"AngleRange\":70,\r\n                                    \"AngleTolerance\":1,\r\n                                    \"StepSize\":3,\r\n                                    \"MinSNR\":0,\r\n                                    \"MinPoints\":25,\r\n                                    \"HoughIterations\":5\r\n                                },\r\n                                \"SearchDirection\":2\r\n                            },\r\n                            \"Measurement\":{\r\n                                \"ROI1\":{\r\n                                    \"Enable\":true,\r\n                                    \"ROI\":{\r\n                                        \"Left\":320,\r\n                                        \"Top\":200,\r\n                                        \"Right\":330,\r\n                                        \"Bottom\":600,\r\n                                        \"Rotation\":0\r\n                                    },\r\n                                    \"EdgeOptions\":{\r\n                                        \"EdgePoarity\":0,\r\n                                        \"KernelSize\":5,\r\n                                        \"Width\":5,\r\n                                        \"MinimumEdgeStrength\":50,\r\n                                        \"InterpolationType\":0,\r\n                                        \"DataProcessingMethod\":0\r\n                                    },\r\n                                    \"LineOptions\":{\r\n                                        \"NumberofLines\":1,\r\n                                        \"Type\":1,\r\n                                        \"MinScore\":10,\r\n                                        \"MaxScore\":1000,\r\n                                        \"Orientation\":0,\r\n                                        \"AngleRange\":30,\r\n                                        \"AngleTolerance\":1,\r\n                                        \"StepSize\":3,\r\n                                        \"MinSNR\":0,\r\n                                        \"MinPoints\":25,\r\n                                        \"HoughIterations\":5\r\n                                    },\r\n                                    \"Process\":1,\r\n                                    \"StepSize\":3,\r\n                                    \"SearchDirection\":2,\r\n                                    \"CircleEdgeOptions\":{\r\n                                        \"SearchDirection\":0,\r\n                                        \"EdgeOptions\":{\r\n                                            \"EdgePoarity\":2,\r\n                                            \"KernelSize\":5,\r\n                                            \"Width\":5,\r\n                                            \"MinimumEdgeStrength\":50,\r\n                                            \"InterpolationType\":1,\r\n                                            \"DataProcessingMethod\":1\r\n                                        }\r\n                                    },\r\n                                    \"CircleFitOptions\":{\r\n                                        \"Process\":3,\r\n                                        \"StepSize\":3,\r\n                                        \"MAxPixelRadius\":3.8500000000000000000\r\n                                    },\r\n                                    \"CircleSearchDirection\":1,\r\n                                    \"CurveParameters\":{\r\n                                        \"ExtractionMode\":0,\r\n                                        \"EdgeThreshold\":50,\r\n                                        \"EdgeFilterSize\":0,\r\n                                        \"MinLength\":25,\r\n                                        \"RowSearchStepSize\":15,\r\n                                        \"ColSearchStepSize\":15,\r\n                                        \"MaxEndpointGap\":10,\r\n                                        \"Closed\":true,\r\n                                        \"Subpixel\":true\r\n                                    },\r\n                                    \"MinimumMatchScore\":800,\r\n                                    \"CircleDescriptor\":{\r\n                                        \"MinRadius\":3,\r\n                                        \"MaxRadius\":200\r\n                                    },\r\n                                    \"EllipseDescriptor\":{\r\n                                        \"MinMajorRadius\":2,\r\n                                        \"MaxMajorRadius\":200,\r\n                                        \"MinMinorRadius\":2,\r\n                                        \"MaxMinorRadius\":100\r\n                                    }\r\n                                },\r\n                                \"ROI2\":{\r\n                                    \"Enable\":false,\r\n                                    \"ROI\":{\r\n                                        \"Left\":739,\r\n                                        \"Top\":305,\r\n                                        \"Right\":763,\r\n                                        \"Bottom\":538,\r\n                                        \"Rotation\":0\r\n                                    },\r\n                                    \"EdgeOptions\":{\r\n                                        \"EdgePoarity\":0,\r\n                                        \"KernelSize\":5,\r\n                                        \"Width\":5,\r\n                                        \"MinimumEdgeStrength\":50,\r\n                                        \"InterpolationType\":0,\r\n                                        \"DataProcessingMethod\":0\r\n                                    },\r\n                                    \"LineOptions\":{\r\n                                        \"NumberofLines\":1,\r\n                                        \"Type\":1,\r\n                                        \"MinScore\":10,\r\n                                        \"MaxScore\":1000,\r\n                                        \"Orientation\":0,\r\n                                        \"AngleRange\":30,\r\n                                        \"AngleTolerance\":1,\r\n                                        \"StepSize\":3,\r\n                                        \"MinSNR\":0,\r\n                                        \"MinPoints\":25,\r\n                                        \"HoughIterations\":5\r\n                                    },\r\n                                    \"Process\":1,\r\n                                    \"StepSize\":2,\r\n                                    \"SearchDirection\":2,\r\n                                    \"CircleEdgeOptions\":{\r\n                                        \"SearchDirection\":0,\r\n                                        \"EdgeOptions\":{\r\n                                            \"EdgePoarity\":2,\r\n                                            \"KernelSize\":3,\r\n                                            \"Width\":3,\r\n                                            \"MinimumEdgeStrength\":50,\r\n                                            \"InterpolationType\":1,\r\n                                            \"DataProcessingMethod\":1\r\n                                        }\r\n                                    },\r\n                                    \"CircleFitOptions\":{\r\n                                        \"Process\":3,\r\n                                        \"StepSize\":3,\r\n                                        \"MAxPixelRadius\":3.8500000000000000000\r\n                                    },\r\n                                    \"CircleSearchDirection\":1,\r\n                                    \"CurveParameters\":{\r\n                                        \"ExtractionMode\":0,\r\n                                        \"EdgeThreshold\":50,\r\n                                        \"EdgeFilterSize\":0,\r\n                                        \"MinLength\":25,\r\n                                        \"RowSearchStepSize\":15,\r\n                                        \"ColSearchStepSize\":15,\r\n                                        \"MaxEndpointGap\":10,\r\n                                        \"Closed\":true,\r\n                                        \"Subpixel\":true\r\n                                    },\r\n                                    \"MinimumMatchScore\":800,\r\n                                    \"CircleDescriptor\":{\r\n                                        \"MinRadius\":3,\r\n                                        \"MaxRadius\":200\r\n                                    },\r\n                                    \"EllipseDescriptor\":{\r\n                                        \"MinMajorRadius\":2,\r\n                                        \"MaxMajorRadius\":200,\r\n                                        \"MinMinorRadius\":2,\r\n                                        \"MaxMinorRadius\":100\r\n                                    }\r\n                                }\r\n                            }\r\n                        },\r\n                        \"MathExpression\":{\r\n                            \"Algorithm\":\"Default\",\r\n                            \"MathExpression\":\"c = 1*c + 0\",\r\n                            \"ResultVariable\":\"c\"\r\n                        },\r\n                        \"MathCorrectionParameters\":{\r\n                            \"Radius\":1.1000000000000000000,\r\n                            \"CurlGap\":0.90000000000000000000,\r\n                            \"Thickness\":0.32000000000000000000,\r\n                            \"MeasurementIndices\":[\r\n                                1\r\n                            ],\r\n                            \"MathAlgoName\":\"Test\",\r\n                            \"MathAlgoFormula\":\"Test2\",\r\n                            \"CorrectionForAngle\":[\r\n                                -2\r\n                            ],\r\n                            \"NumericAray\":[\r\n                                1.1000000000000000000\r\n                            ],\r\n                            \"StringArray\":[\r\n                                \"Test\"\r\n                            ]\r\n                        },\r\n                        \"ResultVariableCluster\":{\r\n                            \"RVName\":\"c\",\r\n                            \"RVSequence\":\"MeasROI1\",\r\n                            \"RVIndex\":1,\r\n                            \"RVID\":1,\r\n                            \"RVValue\":22.600000000000000000\r\n                        },\r\n                        \"CalibrationCoefficients\":{\r\n                            \"A1\":1.6800000000000000000,\r\n                            \"A2\":1.7800000000000000000,\r\n                            \"A3\":1.7600000000000000000\r\n                        },\r\n                        \"UserCalibCoefficients\":{\r\n                            \"UserCorrectionLinearityCoeff\":0.80000000000000000000,\r\n                            \"UserCorrectionBiasCoeff\":0.44300000000000000000\r\n                        },\r\n                        \"SpecValues\":{\r\n                            \"LCL\":2.1500000000000000000,\r\n                            \"UCL\":2.3500000000000000000,\r\n                            \"LSL\":2.1500000000000000000,\r\n                            \"USL\":2.3500000000000000000,\r\n                            \"NominalValue\":2.2500000000000000000\r\n                        },\r\n                        \"OverlayOptions\":{\r\n                            \"OverlayEnable\":true,\r\n                            \"OverlayText\":\"Width\",\r\n                            \"OverlayCoords\":[\r\n                                5,\r\n                                8\r\n                            ],\r\n                            \"OverlayAngle\":56,\r\n                            \"OverlayTextSize\":6,\r\n                            \"OverlayTextColor\":\"Blue\",\r\n                            \"OverlayROI\":true,\r\n                            \"OverlayRakeLine\":true,\r\n                            \"OverlayPoints\":true\r\n                        },\r\n                        \"DatalogEnable\":true,\r\n                        \"DisplayIcon\":\"C:\\\\Desktop\\\\displayimage.png\"\r\n                    }\r\n                ]\r\n            }\r\n        ],\r\n        \"AlgoDefaultParameters\":{\r\n            \"AlgoName\":\"MaxClamp\",\r\n            \"Enable\":true,\r\n            \"AlgorithmSequenceDefault\":{\r\n                \"RefernceEdgeDefault\":{\r\n                    \"Method\":\"LineFinding\",\r\n                    \"RefROI\":{\r\n                        \"Left\":1014,\r\n                        \"Top\":95,\r\n                        \"Right\":1290,\r\n                        \"Bottom\":520,\r\n                        \"Rotation\":0\r\n                    },\r\n                    \"EdgeOptions\":{\r\n                        \"EdgePoarity\":0,\r\n                        \"KernelSize\":3,\r\n                        \"Width\":3,\r\n                        \"MinimumEdgeStrength\":50,\r\n                        \"InterpolationType\":1,\r\n                        \"DataProcessingMethod\":1\r\n                    },\r\n                    \"LineOptions\":{\r\n                        \"NumberofLines\":1,\r\n                        \"Type\":1,\r\n                        \"MinScore\":10,\r\n                        \"MaxScore\":1000,\r\n                        \"Orientation\":0,\r\n                        \"AngleRange\":10,\r\n                        \"AngleTolerance\":1,\r\n                        \"StepSize\":3,\r\n                        \"MinSNR\":0,\r\n                        \"MinPoints\":25,\r\n                        \"HoughIterations\":5\r\n                    },\r\n                    \"SearchDirection\":2\r\n                },\r\n                \"MeasurementDefault\":{\r\n                    \"ROI1\":{\r\n                        \"ROI\":{\r\n                            \"Left\":100,\r\n                            \"Top\":150,\r\n                            \"Right\":400,\r\n                            \"Bottom\":700,\r\n                            \"Rotation\":0\r\n                        },\r\n                        \"EdgeOptions\":{\r\n                            \"EdgePoarity\":0,\r\n                            \"KernelSize\":3,\r\n                            \"Width\":3,\r\n                            \"MinimumEdgeStrength\":50,\r\n                            \"InterpolationType\":1,\r\n                            \"DataProcessingMethod\":1\r\n                        },\r\n                        \"LineOptions\":{\r\n                            \"NumberofLines\":1,\r\n                            \"Type\":1,\r\n                            \"MinScore\":10,\r\n                            \"MaxScore\":1000,\r\n                            \"Orientation\":0,\r\n                            \"AngleRange\":10,\r\n                            \"AngleTolerance\":1,\r\n                            \"StepSize\":3,\r\n                            \"MinSNR\":0,\r\n                            \"MinPoints\":25,\r\n                            \"HoughIterations\":5\r\n                        },\r\n                        \"Process\":1,\r\n                        \"StepSize\":10,\r\n                        \"SearchDirection\":0,\r\n                        \"CircleEdgeOptions\":{\r\n                            \"SearchDirection\":1,\r\n                            \"EdgeOptions\":{\r\n                                \"EdgePoarity\":0,\r\n                                \"KernelSize\":3,\r\n                                \"Width\":3,\r\n                                \"MinimumEdgeStrength\":50,\r\n                                \"InterpolationType\":1,\r\n                                \"DataProcessingMethod\":1\r\n                            }\r\n                        },\r\n                        \"CircleFitOptions\":{\r\n                            \"Process\":3,\r\n                            \"StepSize\":3,\r\n                            \"MAxPixelRadius\":3\r\n                        },\r\n                        \"CircleSearchDirection\":1,\r\n                        \"CurveParameters\":{\r\n                            \"ExtractionMode\":0,\r\n                            \"EdgeThreshold\":50,\r\n                            \"EdgeFilterSize\":0,\r\n                            \"MinLength\":25,\r\n                            \"RowSearchStepSize\":15,\r\n                            \"ColSearchStepSize\":15,\r\n                            \"MaxEndpointGap\":10,\r\n                            \"Closed\":0,\r\n                            \"Subpixel\":0\r\n                        },\r\n                        \"MinimumMatchScore\":800,\r\n                        \"CircleDescriptor\":{\r\n                            \"MinRadius\":3,\r\n                            \"MaxRadius\":200\r\n                        },\r\n                        \"EllipseDescriptor\":{\r\n                            \"MinMajorRadius\":2,\r\n                            \"MaxMajorRadius\":200,\r\n                            \"MinMinorRadius\":2,\r\n                            \"MaxMinorRadius\":100\r\n                        },\r\n                        \"OverlayOptions\":{\r\n                            \"OverlayEnable\":true,\r\n                            \"OverlayText\":\"Collar Width\",\r\n                            \"OverlayCoords\":[\r\n                                5,\r\n                                8\r\n                            ],\r\n                            \"OverlayAngle\":56,\r\n                            \"OverlayTextSize\":6,\r\n                            \"OverlayTextColor\":\"Red\"\r\n                        },\r\n                        \"ResultVariable\":\"M1\"\r\n                    },\r\n                    \"ROI2\":{\r\n                        \"ROI\":{\r\n                            \"Left\":100,\r\n                            \"Top\":150,\r\n                            \"Right\":400,\r\n                            \"Bottom\":700,\r\n                            \"Rotation\":0\r\n                        },\r\n                        \"EdgeOptions\":{\r\n                            \"EdgePoarity\":0,\r\n                            \"KernelSize\":3,\r\n                            \"Width\":3,\r\n                            \"MinimumEdgeStrength\":50,\r\n                            \"InterpolationType\":1,\r\n                            \"DataProcessingMethod\":1\r\n                        },\r\n                        \"LineOptions\":{\r\n                            \"NumberofLines\":1,\r\n                            \"Type\":1,\r\n                            \"MinScore\":10,\r\n                            \"MaxScore\":1000,\r\n                            \"Orientation\":0,\r\n                            \"AngleRange\":10,\r\n                            \"AngleTolerance\":1,\r\n                            \"StepSize\":3,\r\n                            \"MinSNR\":0,\r\n                            \"MinPoints\":25,\r\n                            \"HoughIterations\":5\r\n                        },\r\n                        \"Process\":1,\r\n                        \"StepSize\":10,\r\n                        \"SearchDirection\":0,\r\n                        \"CircleEdgeOptions\":{\r\n                            \"SearchDirection\":1,\r\n                            \"EdgeOptions\":{\r\n                                \"EdgePoarity\":0,\r\n                                \"KernelSize\":3,\r\n                                \"Width\":3,\r\n                                \"MinimumEdgeStrength\":50,\r\n                                \"InterpolationType\":1,\r\n                                \"DataProcessingMethod\":1\r\n                            }\r\n                        },\r\n                        \"CircleFitOptions\":{\r\n                            \"Process\":3,\r\n                            \"StepSize\":3,\r\n                            \"MaxPixelRadius\":3\r\n                        },\r\n                        \"CircleSearchDirection\":1,\r\n                        \"CurveParameters\":{\r\n                            \"ExtractionMode\":0,\r\n                            \"EdgeThreshold\":50,\r\n                            \"EdgeFilterSize\":0,\r\n                            \"MinLength\":25,\r\n                            \"RowSearchStepSize\":15,\r\n                            \"ColSearchStepSize\":15,\r\n                            \"MaxEndpointGap\":10,\r\n                            \"Closed\":0,\r\n                            \"Subpixel\":0\r\n                        },\r\n                        \"MinimumMatchScore\":800,\r\n                        \"CircleDescriptor\":{\r\n                            \"MinRadius\":3,\r\n                            \"MaxRadius\":200\r\n                        },\r\n                        \"EllipseDescriptor\":{\r\n                            \"MinMajorRadius\":2,\r\n                            \"MaxMajorRadius\":200,\r\n                            \"MinMinorRadius\":2,\r\n                            \"MaxMinorRadius\":100\r\n                        },\r\n                        \"OverlayOptions\":{\r\n                            \"OverlayEnable\":true,\r\n                            \"OverlayText\":\"Collar Width\",\r\n                            \"OverlayCoords\":[\r\n                                5,\r\n                                8\r\n                            ],\r\n                            \"OverlayAngle\":56,\r\n                            \"OverlayTextSize\":6,\r\n                            \"OverlayTextColor\":\"Red\"\r\n                        },\r\n                        \"ResultVariable\":\"M2\"\r\n                    }\r\n                },\r\n                \"MathExpressionDefault\":{\r\n                    \"Algorithm\":\"Math1\",\r\n                    \"MathExpression\":\"M2-M1\",\r\n                    \"ResultVariable\":\"M3\"\r\n                }\r\n            },\r\n            \"CalibrationCoefficients\":{\r\n                \"A1\":13,\r\n                \"A2\":8.7000000000000000000,\r\n                \"A3\":67.900000000000000000\r\n            },\r\n            \"UserCalibCoefficients\":{\r\n                \"UserCorrectionBiasCoeff\":56,\r\n                \"UserCorrectionLinearityCoeff\":45\r\n            },\r\n            \"OverlayOptions\":{\r\n                \"OverlayEnable\":true,\r\n                \"OverlayText\":\"Collar Width\",\r\n                \"OverlayCoords\":[\r\n                    5,\r\n                    8\r\n                ],\r\n                \"OverlayAngle\":23,\r\n                \"OverlayTextSize\":6,\r\n                \"OverlayTextColor\":\"Red\"\r\n            },\r\n            \"DatalogEnable\":true,\r\n            \"DisplayIcon\":\"C:\\\\Desktop\\\\displayimage.png\"\r\n        }\r\n    }\r\n}", 11 "Reference structure":string="{\n    \"SpecificationVersion\":\"\",\n    \"CompatibleSoftwareVersions\":[\n        \"trt\"\n    ],\n    \"AlgoParameters\":{\n        \"PartsList\":[\n            {\n                \"Name\":\"\",\n                \"ImageStreams\":[\n                    {\n                        \"ThreadName\":\"\",\n                        \"RackEnable\":false,\n                        \"ThreadId\":0.00000000000000,\n                        \"RackId\":0.00000000000000,\n                        \"DifferenceParameter\":0.00000000000000,\n                        \"SplitCameraIDs\":[\n                            3\n                        ],\n                        \"ImagingViews\":[\n                            {\n                                \"ViewName\":\"\",\n                                \"ViewEnable\":false,\n                                \"ImageID\":0.00000000000000,\n                                \"CameraID\":0.00000000000000,\n                                \"CalibrationFilePath\":\"\",\n                                \"CalibImageFormat\":\"\",\n                                \"ReferenceCoordSystem\":{\n                                    \"Method\":{\n                                        \"Algo\":\"\",\n                                        \"BaseReference\":{\n                                            \"OriginX\":0.00000000000000,\n                                            \"OriginY\":0.00000000000000,\n                                            \"Angle\":0.00000000000000,\n                                            \"AxisReference\":0.00000000000000\n                                        }\n                                    },\n                                    \"ROI\":[\n                                        {\n                                            \"ROI\":{\n                                                \"Left\":0.00000000000000,\n                                                \"Top\":0.00000000000000,\n                                                \"Right\":0.00000000000000,\n                                                \"Bottom\":0.00000000000000,\n                                                \"Rotation\":0.00000000000000\n                                            },\n                                            \"EdgeOptions\":{\n                                                \"EdgePolarity\":0.00000000000000,\n                                                \"KernelSize\":0.00000000000000,\n                                                \"Width\":0.00000000000000,\n                                                \"MinimumEdgeStrength\":0.00000000000000,\n                                                \"InterpolationType\":0.00000000000000,\n                                                \"DataProcessingMethod\":0.00000000000000\n                                            },\n                                            \"LineOptions\":{\n                                                \"NumberofLines\":0.00000000000000,\n                                                \"Type\":0.00000000000000,\n                                                \"MinScore\":0.00000000000000,\n                                                \"MaxScore\":0.00000000000000,\n                                                \"Orientation\":0.00000000000000,\n                                                \"AngleRange\":0.00000000000000,\n                                                \"AngleTolerance\":0.00000000000000,\n                                                \"StepSize\":0.00000000000000,\n                                                \"MinSNR\":0.00000000000000,\n                                                \"MinPoints\":0.00000000000000,\n                                                \"HoughIterations\":0.00000000000000\n                                            },\n                                            \"Process\":0.00000000000000,\n                                            \"StepSize\":0.00000000000000,\n                                            \"SearchDirection\":0.00000000000000,\n                                            \"CircleEdgeOptions\":{\n                                                \"SearchDirection\":0.00000000000000,\n                                                \"EdgeOptions\":{\n                                                    \"EdgePolarity\":0.00000000000000,\n                                                    \"KernelSize\":0.00000000000000,\n                                                    \"Width\":0.00000000000000,\n                                                    \"MinimumEdgeStrength\":0.00000000000000,\n                                                    \"InterpolationType\":0.00000000000000,\n                                                    \"DataProcessingMethod\":0.00000000000000\n                                                }\n                                            },\n                                            \"CircleFitOptions\":{\n                                                \"Process\":0.00000000000000,\n                                                \"StepSize\":0.00000000000000,\n                                                \"MAxPixelRadius\":0.00000000000000\n                                            },\n                                            \"CircleSearchDirection\":0.00000000000000,\n                                            \"CurveParameters\":{\n                                                \"ExtractionMode\":0.00000000000000,\n                                                \"EdgeThreshold\":0.00000000000000,\n                                                \"EdgeFilterSize\":0.00000000000000,\n                                                \"MinLength\":0.00000000000000,\n                                                \"RowSearchStepSize\":0.00000000000000,\n                                                \"ColSearchStepSize\":0.00000000000000,\n                                                \"MaxEndpointGap\":0.00000000000000,\n                                                \"Closed\":false,\n                                                \"Subpixel\":false\n                                            },\n                                            \"MinimumMatchScore\":0.00000000000000,\n                                            \"CircleDescriptor\":{\n                                                \"MinRadius\":5.00000000000000,\n                                                \"MaxRadius\":0.00000000000000\n                                            },\n                                            \"EllipseDescriptor\":{\n                                                \"MinMajorRadius\":0.00000000000000,\n                                                \"MaxMajorRadius\":0.00000000000000,\n                                                \"MinMinorRadius\":0.00000000000000,\n                                                \"MaxMinorRadius\":0.00000000000000\n                                            },\n                                            \"ParallelLines\":{\n                                                \"First\":0.00000000000000,\n                                                \"Second\":0.00000000000000,\n                                                \"Third\":0.00000000000000\n                                            }\n                                        }\n                                    ],\n                                    \"Name\":\"\",\n                                    \"OverlayOptions\":{\n                                        \"OverlayEnable\":false,\n                                        \"OverlayText\":\"\",\n                                        \"OverlayCoords\":[\n                                            5\n                                        ],\n                                        \"OverlayAngle\":0.00000000000000,\n                                        \"OverlayTextSize\":0.00000000000000,\n                                        \"OverlayTextColor\":\"\",\n                                        \"OverlayROI\":false,\n                                        \"OverlayRakeLine\":false,\n                                        \"OverlayPoints\":false\n                                    }\n                                },\n                                \"CameraAngle\":[\n                                    5\n                                ]\n                            }\n                        ]\n                    }\n                ],\n                \"Measurements\":[\n                    {\n                        \"RackID\":0.00000000000000,\n                        \"ImageID\":0.00000000000000,\n                        \"CameraID\":0.00000000000000,\n                        \"MeasurementId\":0.00000000000000,\n                        \"Name\":\"\",\n                        \"AlgoName\":\"\",\n                        \"Type\":\"\",\n                        \"MeasurementEnable\":false,\n                        \"AlgorithmSequence\":{\n                            \"RefernceEdge\":{\n                                \"Enable\":false,\n                                \"Method\":\"\",\n                                \"RefROI\":{\n                                    \"Left\":0.00000000000000,\n                                    \"Top\":0.00000000000000,\n                                    \"Right\":0.00000000000000,\n                                    \"Bottom\":0.00000000000000,\n                                    \"Rotation\":0.00000000000000\n                                },\n                                \"EdgeOptions\":{\n                                    \"EdgePoarity\":0.00000000000000,\n                                    \"KernelSize\":0.00000000000000,\n                                    \"Width\":0.00000000000000,\n                                    \"MinimumEdgeStrength\":0.00000000000000,\n                                    \"InterpolationType\":0.00000000000000,\n                                    \"DataProcessingMethod\":0.00000000000000\n                                },\n                                \"LineOptions\":{\n                                    \"NumberofLines\":0.00000000000000,\n                                    \"Type\":0.00000000000000,\n                                    \"MinScore\":0.00000000000000,\n                                    \"MaxScore\":0.00000000000000,\n                                    \"Orientation\":0.00000000000000,\n                                    \"AngleRange\":0.00000000000000,\n                                    \"AngleTolerance\":0.00000000000000,\n                                    \"StepSize\":0.00000000000000,\n                                    \"MinSNR\":0.00000000000000,\n                                    \"MinPoints\":0.00000000000000,\n                                    \"HoughIterations\":0.00000000000000\n                                },\n                                \"SearchDirection\":0.00000000000000\n                            },\n                            \"Measurement\":{\n                                \"ROI1\":{\n                                    \"Enable\":false,\n                                    \"ROI\":{\n                                        \"Left\":0.00000000000000,\n                                        \"Top\":0.00000000000000,\n                                        \"Right\":0.00000000000000,\n                                        \"Bottom\":0.00000000000000,\n                                        \"Rotation\":0.00000000000000\n                                    },\n                                    \"EdgeOptions\":{\n                                        \"EdgePoarity\":0.00000000000000,\n                                        \"KernelSize\":0.00000000000000,\n                                        \"Width\":0.00000000000000,\n                                        \"MinimumEdgeStrength\":0.00000000000000,\n                                        \"InterpolationType\":0.00000000000000,\n                                        \"DataProcessingMethod\":0.00000000000000\n                                    },\n                                    \"LineOptions\":{\n                                        \"NumberofLines\":0.00000000000000,\n                                        \"Type\":0.00000000000000,\n                                        \"MinScore\":0.00000000000000,\n                                        \"MaxScore\":0.00000000000000,\n                                        \"Orientation\":0.00000000000000,\n                                        \"AngleRange\":0.00000000000000,\n                                        \"AngleTolerance\":0.00000000000000,\n                                        \"StepSize\":0.00000000000000,\n                                        \"MinSNR\":0.00000000000000,\n                                        \"MinPoints\":0.00000000000000,\n                                        \"HoughIterations\":0.00000000000000\n                                    },\n                                    \"Process\":0.00000000000000,\n                                    \"StepSize\":0.00000000000000,\n                                    \"SearchDirection\":0.00000000000000,\n                                    \"CircleEdgeOptions\":{\n                                        \"SearchDirection\":0.00000000000000,\n                                        \"EdgeOptions\":{\n                                            \"EdgePoarity\":0.00000000000000,\n                                            \"KernelSize\":0.00000000000000,\n                                            \"Width\":0.00000000000000,\n                                            \"MinimumEdgeStrength\":0.00000000000000,\n                                            \"InterpolationType\":0.00000000000000,\n                                            \"DataProcessingMethod\":0.00000000000000\n                                        }\n                                    },\n                                    \"CircleFitOptions\":{\n                                        \"Process\":0.00000000000000,\n                                        \"StepSize\":0.00000000000000,\n                                        \"MAxPixelRadius\":0.00000000000000\n                                    },\n                                    \"CircleSearchDirection\":0.00000000000000,\n                                    \"CurveParameters\":{\n                                        \"ExtractionMode\":0.00000000000000,\n                                        \"EdgeThreshold\":0.00000000000000,\n                                        \"EdgeFilterSize\":0.00000000000000,\n                                        \"MinLength\":0.00000000000000,\n                                        \"RowSearchStepSize\":0.00000000000000,\n                                        \"ColSearchStepSize\":0.00000000000000,\n                                        \"MaxEndpointGap\":0.00000000000000,\n                                        \"Closed\":false,\n                                        \"Subpixel\":false\n                                    },\n                                    \"MinimumMatchScore\":0.00000000000000,\n                                    \"CircleDescriptor\":{\n                                        \"MinRadius\":0.00000000000000,\n                                        \"MaxRadius\":0.00000000000000\n                                    },\n                                    \"EllipseDescriptor\":{\n                                        \"MinMajorRadius\":0.00000000000000,\n                                        \"MaxMajorRadius\":0.00000000000000,\n                                        \"MinMinorRadius\":0.00000000000000,\n                                        \"MaxMinorRadius\":0.00000000000000\n                                    }\n                                },\n                                \"ROI2\":{\n                                    \"Enable\":false,\n                                    \"ROI\":{\n                                        \"Left\":0.00000000000000,\n                                        \"Top\":0.00000000000000,\n                                        \"Right\":0.00000000000000,\n                                        \"Bottom\":0.00000000000000,\n                                        \"Rotation\":0.00000000000000\n                                    },\n                                    \"EdgeOptions\":{\n                                        \"EdgePoarity\":0.00000000000000,\n                                        \"KernelSize\":0.00000000000000,\n                                        \"Width\":0.00000000000000,\n                                        \"MinimumEdgeStrength\":0.00000000000000,\n                                        \"InterpolationType\":0.00000000000000,\n                                        \"DataProcessingMethod\":0.00000000000000\n                                    },\n                                    \"LineOptions\":{\n                                        \"NumberofLines\":0.00000000000000,\n                                        \"Type\":0.00000000000000,\n                                        \"MinScore\":0.00000000000000,\n                                        \"MaxScore\":0.00000000000000,\n                                        \"Orientation\":0.00000000000000,\n                                        \"AngleRange\":0.00000000000000,\n                                        \"AngleTolerance\":0.00000000000000,\n                                        \"StepSize\":0.00000000000000,\n                                        \"MinSNR\":0.00000000000000,\n                                        \"MinPoints\":0.00000000000000,\n                                        \"HoughIterations\":0.00000000000000\n                                    },\n                                    \"Process\":0.00000000000000,\n                                    \"StepSize\":0.00000000000000,\n                                    \"SearchDirection\":0.00000000000000,\n                                    \"CircleEdgeOptions\":{\n                                        \"SearchDirection\":0.00000000000000,\n                                        \"EdgeOptions\":{\n                                            \"EdgePoarity\":0.00000000000000,\n                                            \"KernelSize\":0.00000000000000,\n                                            \"Width\":0.00000000000000,\n                                            \"MinimumEdgeStrength\":0.00000000000000,\n                                            \"InterpolationType\":0.00000000000000,\n                                            \"DataProcessingMethod\":0.00000000000000\n                                        }\n                                    },\n                                    \"CircleFitOptions\":{\n                                        \"Process\":0.00000000000000,\n                                        \"StepSize\":0.00000000000000,\n                                        \"MAxPixelRadius\":0.00000000000000\n                                    },\n                                    \"CircleSearchDirection\":0.00000000000000,\n                                    \"CurveParameters\":{\n                                        \"ExtractionMode\":0.00000000000000,\n                                        \"EdgeThreshold\":0.00000000000000,\n                                        \"EdgeFilterSize\":0.00000000000000,\n                                        \"MinLength\":0.00000000000000,\n                                        \"RowSearchStepSize\":0.00000000000000,\n                                        \"ColSearchStepSize\":0.00000000000000,\n                                        \"MaxEndpointGap\":0.00000000000000,\n                                        \"Closed\":false,\n                                        \"Subpixel\":false\n                                    },\n                                    \"MinimumMatchScore\":0.00000000000000,\n                                    \"CircleDescriptor\":{\n                                        \"MinRadius\":0.00000000000000,\n                                        \"MaxRadius\":0.00000000000000\n                                    },\n                                    \"EllipseDescriptor\":{\n                                        \"MinMajorRadius\":0.00000000000000,\n                                        \"MaxMajorRadius\":0.00000000000000,\n                                        \"MinMinorRadius\":0.00000000000000,\n                                        \"MaxMinorRadius\":0.00000000000000\n                                    }\n                                }\n                            }\n                        },\n                        \"MathExpression\":{\n                            \"Algorithm\":\"\",\n                            \"MathExpression\":\"\",\n                            \"ResultVariable\":\"\"\n                        },\n                        \"MathCorrectionParameters\":{\n                            \"Radius\":0.00000000000000,\n                            \"CurlGap\":0.00000000000000,\n                            \"Thickness\":0.00000000000000,\n                            \"MeasurementIndices\":[\n                                5\n                            ],\n                            \"MathAlgoName\":\"\",\n                            \"MathAlgoFormula\":\"\",\n                            \"CorrectionForAngle\":[\n                                35\n                            ],\n                            \"NumericAray\":[\n                                0\n                            ],\n                            \"StringArray\":[\n                                \"gfdgf\"\n                            ]\n                        },\n                        \"ResultVariableCluster\":{\n                            \"RVName\":\"\",\n                            \"RVSequence\":\"\",\n                            \"RVIndex\":0.00000000000000,\n                            \"RVID\":0.00000000000000,\n                            \"RVValue\":0.00000000000000\n                        },\n                        \"CalibrationCoefficients\":{\n                            \"A1\":0.00000000000000,\n                            \"A2\":0.00000000000000,\n                            \"A3\":0.00000000000000\n                        },\n                        \"UserCalibCoefficients\":{\n                            \"UserCorrectionLinearityCoeff\":0.00000000000000,\n                            \"UserCorrectionBiasCoeff\":0.00000000000000\n                        },\n                        \"SpecValues\":{\n                            \"LCL\":0.00000000000000,\n                            \"UCL\":0.00000000000000,\n                            \"LSL\":0.00000000000000,\n                            \"USL\":0.00000000000000,\n                            \"NominalValue\":0.00000000000000\n                        },\n                        \"OverlayOptions\":{\n                            \"OverlayEnable\":false,\n                            \"OverlayText\":\"\",\n                            \"OverlayCoords\":[\n                                3\n                            ],\n                            \"OverlayAngle\":0.00000000000000,\n                            \"OverlayTextSize\":0.00000000000000,\n                            \"OverlayTextColor\":\"\",\n                            \"OverlayROI\":false,\n                            \"OverlayRakeLine\":false,\n                            \"OverlayPoints\":false\n                        },\n                        \"DatalogEnable\":false,\n                        \"DisplayIcon\":\"test\"\n                    }\n                ]\n            }\n        ],\n        \"AlgoDefaultParameters\":{\n            \"AlgoName\":\"\",\n            \"Enable\":false,\n            \"AlgorithmSequenceDefault\":{\n                \"RefernceEdgeDefault\":{\n                    \"Method\":\"\",\n                    \"RefROI\":{\n                        \"Left\":0.00000000000000,\n                        \"Top\":0.00000000000000,\n                        \"Right\":0.00000000000000,\n                        \"Bottom\":0.00000000000000,\n                        \"Rotation\":0.00000000000000\n                    },\n                    \"EdgeOptions\":{\n                        \"EdgePoarity\":0.00000000000000,\n                        \"KernelSize\":0.00000000000000,\n                        \"Width\":0.00000000000000,\n                        \"MinimumEdgeStrength\":0.00000000000000,\n                        \"InterpolationType\":0.00000000000000,\n                        \"DataProcessingMethod\":0.00000000000000\n                    },\n                    \"LineOptions\":{\n                        \"NumberofLines\":0.00000000000000,\n                        \"Type\":0.00000000000000,\n                        \"MinScore\":0.00000000000000,\n                        \"MaxScore\":0.00000000000000,\n                        \"Orientation\":0.00000000000000,\n                        \"AngleRange\":0.00000000000000,\n                        \"AngleTolerance\":0.00000000000000,\n                        \"StepSize\":0.00000000000000,\n                        \"MinSNR\":0.00000000000000,\n                        \"MinPoints\":0.00000000000000,\n                        \"HoughIterations\":0.00000000000000\n                    },\n                    \"SearchDirection\":0.00000000000000\n                },\n                \"MeasurementDefault\":{\n                    \"ROI1\":{\n                        \"ROI\":{\n                            \"Left\":0.00000000000000,\n                            \"Top\":0.00000000000000,\n                            \"Right\":0.00000000000000,\n                            \"Bottom\":0.00000000000000,\n                            \"Rotation\":0.00000000000000\n                        },\n                        \"EdgeOptions\":{\n                            \"EdgePoarity\":0.00000000000000,\n                            \"KernelSize\":0.00000000000000,\n                            \"Width\":0.00000000000000,\n                            \"MinimumEdgeStrength\":0.00000000000000,\n                            \"InterpolationType\":0.00000000000000,\n                            \"DataProcessingMethod\":0.00000000000000\n                        },\n                        \"LineOptions\":{\n                            \"NumberofLines\":0.00000000000000,\n                            \"Type\":0.00000000000000,\n                            \"MinScore\":0.00000000000000,\n                            \"MaxScore\":0.00000000000000,\n                            \"Orientation\":0.00000000000000,\n                            \"AngleRange\":0.00000000000000,\n                            \"AngleTolerance\":0.00000000000000,\n                            \"StepSize\":0.00000000000000,\n                            \"MinSNR\":0.00000000000000,\n                            \"MinPoints\":0.00000000000000,\n                            \"HoughIterations\":0.00000000000000\n                        },\n                        \"Process\":0.00000000000000,\n                        \"StepSize\":0.00000000000000,\n                        \"SearchDirection\":0.00000000000000,\n                        \"CircleEdgeOptions\":{\n                            \"SearchDirection\":0.00000000000000,\n                            \"EdgeOptions\":{\n                                \"EdgePoarity\":0.00000000000000,\n                                \"KernelSize\":0.00000000000000,\n                                \"Width\":0.00000000000000,\n                                \"MinimumEdgeStrength\":0.00000000000000,\n                                \"InterpolationType\":0.00000000000000,\n                                \"DataProcessingMethod\":0.00000000000000\n                            }\n                        },\n                        \"CircleFitOptions\":{\n                            \"Process\":0.00000000000000,\n                            \"StepSize\":0.00000000000000,\n                            \"MAxPixelRadius\":0.00000000000000\n                        },\n                        \"CircleSearchDirection\":0.00000000000000,\n                        \"CurveParameters\":{\n                            \"ExtractionMode\":0.00000000000000,\n                            \"EdgeThreshold\":0.00000000000000,\n                            \"EdgeFilterSize\":0.00000000000000,\n                            \"MinLength\":0.00000000000000,\n                            \"RowSearchStepSize\":0.00000000000000,\n                            \"ColSearchStepSize\":0.00000000000000,\n                            \"MaxEndpointGap\":0.00000000000000,\n                            \"Closed\":0.00000000000000,\n                            \"Subpixel\":0.00000000000000\n                        },\n                        \"MinimumMatchScore\":0.00000000000000,\n                        \"CircleDescriptor\":{\n                            \"MinRadius\":0.00000000000000,\n                            \"MaxRadius\":0.00000000000000\n                        },\n                        \"EllipseDescriptor\":{\n                            \"MinMajorRadius\":0.00000000000000,\n                            \"MaxMajorRadius\":0.00000000000000,\n                            \"MinMinorRadius\":0.00000000000000,\n                            \"MaxMinorRadius\":0.00000000000000\n                        },\n                        \"OverlayOptions\":{\n                            \"OverlayEnable\":false,\n                            \"OverlayText\":\"\",\n                            \"OverlayCoords\":[\n                            ],\n                            \"OverlayAngle\":0.00000000000000,\n                            \"OverlayTextSize\":0.00000000000000,\n                            \"OverlayTextColor\":\"\"\n                        },\n                        \"ResultVariable\":\"\"\n                    },\n                    \"ROI2\":{\n                        \"ROI\":{\n                            \"Left\":0.00000000000000,\n                            \"Top\":0.00000000000000,\n                            \"Right\":0.00000000000000,\n                            \"Bottom\":0.00000000000000,\n                            \"Rotation\":0.00000000000000\n                        },\n                        \"EdgeOptions\":{\n                            \"EdgePoarity\":0.00000000000000,\n                            \"KernelSize\":0.00000000000000,\n                            \"Width\":0.00000000000000,\n                            \"MinimumEdgeStrength\":0.00000000000000,\n                            \"InterpolationType\":0.00000000000000,\n                            \"DataProcessingMethod\":0.00000000000000\n                        },\n                        \"LineOptions\":{\n                            \"NumberofLines\":0.00000000000000,\n                            \"Type\":0.00000000000000,\n                            \"MinScore\":0.00000000000000,\n                            \"MaxScore\":0.00000000000000,\n                            \"Orientation\":0.00000000000000,\n                            \"AngleRange\":0.00000000000000,\n                            \"AngleTolerance\":0.00000000000000,\n                            \"StepSize\":0.00000000000000,\n                            \"MinSNR\":0.00000000000000,\n                            \"MinPoints\":0.00000000000000,\n                            \"HoughIterations\":0.00000000000000\n                        },\n                        \"Process\":0.00000000000000,\n                        \"StepSize\":0.00000000000000,\n                        \"SearchDirection\":0.00000000000000,\n                        \"CircleEdgeOptions\":{\n                            \"SearchDirection\":0.00000000000000,\n                            \"EdgeOptions\":{\n                                \"EdgePoarity\":0.00000000000000,\n                                \"KernelSize\":0.00000000000000,\n                                \"Width\":0.00000000000000,\n                                \"MinimumEdgeStrength\":0.00000000000000,\n                                \"InterpolationType\":0.00000000000000,\n                                \"DataProcessingMethod\":0.00000000000000\n                            }\n                        },\n                        \"CircleFitOptions\":{\n                            \"Process\":0.00000000000000,\n                            \"StepSize\":0.00000000000000,\n                            \"MaxPixelRadius\":0.00000000000000\n                        },\n                        \"CircleSearchDirection\":0.00000000000000,\n                        \"CurveParameters\":{\n                            \"ExtractionMode\":0.00000000000000,\n                            \"EdgeThreshold\":0.00000000000000,\n                            \"EdgeFilterSize\":0.00000000000000,\n                            \"MinLength\":0.00000000000000,\n                            \"RowSearchStepSize\":0.00000000000000,\n                            \"ColSearchStepSize\":0.00000000000000,\n                            \"MaxEndpointGap\":0.00000000000000,\n                            \"Closed\":0.00000000000000,\n                            \"Subpixel\":0.00000000000000\n                        },\n                        \"MinimumMatchScore\":0.00000000000000,\n                        \"CircleDescriptor\":{\n                            \"MinRadius\":0.00000000000000,\n                            \"MaxRadius\":0.00000000000000\n                        },\n                        \"EllipseDescriptor\":{\n                            \"MinMajorRadius\":0.00000000000000,\n                            \"MaxMajorRadius\":0.00000000000000,\n                            \"MinMinorRadius\":0.00000000000000,\n                            \"MaxMinorRadius\":0.00000000000000\n                        },\n                        \"OverlayOptions\":{\n                            \"OverlayEnable\":false,\n                            \"OverlayText\":\"\",\n                            \"OverlayCoords\":[\n                            ],\n                            \"OverlayAngle\":0.00000000000000,\n                            \"OverlayTextSize\":0.00000000000000,\n                            \"OverlayTextColor\":\"\"\n                        },\n                        \"ResultVariable\":\"\"\n                    }\n                },\n                \"MathExpressionDefault\":{\n                    \"Algorithm\":\"\",\n                    \"MathExpression\":\"\",\n                    \"ResultVariable\":\"\"\n                }\n            },\n            \"CalibrationCoefficients\":{\n                \"A1\":0.00000000000000,\n                \"A2\":0.00000000000000,\n                \"A3\":0.00000000000000\n            },\n            \"UserCalibCoefficients\":{\n                \"UserCorrectionBiasCoeff\":0.00000000000000,\n                \"UserCorrectionLinearityCoeff\":0.00000000000000\n            },\n            \"OverlayOptions\":{\n                \"OverlayEnable\":false,\n                \"OverlayText\":\"\",\n                \"OverlayCoords\":[\n                    43\n                ],\n                \"OverlayAngle\":0.00000000000000,\n                \"OverlayTextSize\":0.00000000000000,\n                \"OverlayTextColor\":\"\"\n            },\n            \"DatalogEnable\":false,\n            \"DisplayIcon\":\"\"\n        }\n    }\n}") -> (0 "error out":errorcluster, 3 "Fault element\nJSON path":string)   [LabVIEW 2015]
uses:
  <vilib>/addons/_JKI.lib/Serialization/JSON/JKI JSON Serialization.lvlib
panel:
  out "?":bool
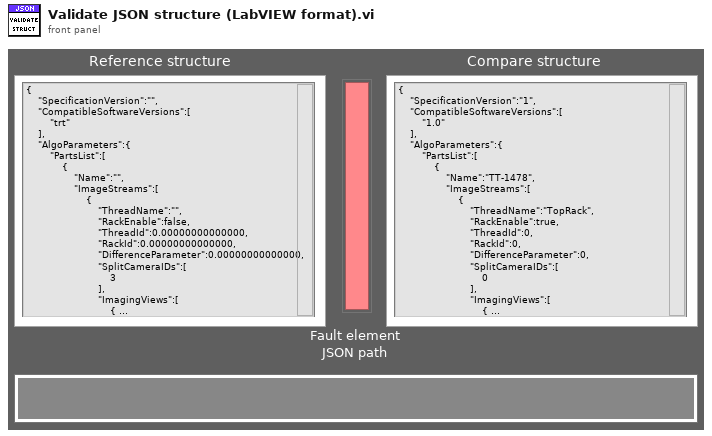
[diagram p1: front panel]
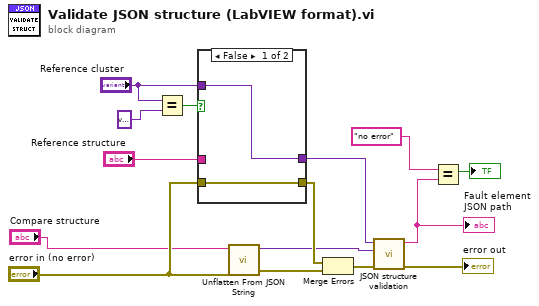
[diagram p0: block diagram]
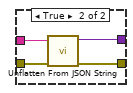
[diagram p2: hidden frame]
diagram:
  n1 = Equal?(x="Reference cluster", y=variant ("Reference cluster")) -> (x = y?=w13:bool)
  n2 = case shown="False" w13 {
    tunnel: "Reference structure" -> [_ w19]
    tunnel: "Reference cluster" -> [w17 _]
    tunnel: [w17 w21] -> w5
    tunnel: "error in (no error)" -> [w16 w20]
    tunnel: [w16 w18] -> w8
    frame False {
    }
    frame True {
      n3 = call <vilib>:"Unflatten From JSON String.vi"("error in (no error)"=w20, "JSON String"=w19) -> ("error out"=w18:errorcluster, "Variant"=w21:variant)  [unwired: 8 in]
    }
  }
  n4 = call <vilib>:"Unflatten From JSON String.vi"("error in (no error)"="error in (no error)", "JSON String"="Compare structure") -> ("error out"=w7:errorcluster, "Variant"=w4:variant)  [unwired: 8 in]
  n5 = Merge Errors(w8, w7) -> (w6:errorcluster)
  n6 = call "JSON structure validation.vi"("error in (no error)"=w6, "Compare\nvariant"=w4, "Reference\nvariant"=w5) -> ("error out"=→"error out":errorcluster, "Element name"=w3:string)  [unwired: 6 in, 1 out]
  "Fault element\nJSON path" <- w3
  n7 = Equal?(x="no error", y=w3) -> (x = y?=→"?":bool)
